vi "Micro-PL v10.6.4.vi"() -> ()   [LabVIEW 2010]
uses:
  drivers/Oxford ITC/ITCAPPS.LLB/ITCSetup.ctl
  drivers/Oxford ITC/ITCSUBS.LLB/ITCIO.ctl
  drivers/Oxford ITC/BUSGEN.LLB/OxfordAddress.ctl
  drivers/Oxford ITC/ITCSUBS.LLB/ITCVersion.ctl
  subvi/NPC3SG/TypeDefs/NPC3SG Live Controls.ctl
  subvi/NPC3SG/TypeDefs/NPC3SG Current Values.ctl
  subvi/NPC3SG/TypeDefs/NPC3SG Set Positions.ctl
  subvi/ITC503/TypeDefs/ITC503 Settings.ctl
  subvi/ITC503/TypeDefs/ITC503 Current Values.ctl
  subvi/iHR550/TypeDefs/iHR Current Values.ctl
  subvi/iHR550/TypeDefs/iHR Settings.ctl
  subvi/Mapping/TypeDefs/Mapping Spectra Params.ctl
  <vilib>/Utility/miscctls.llb/LVBoundsTypeDef.ctl
  subvi/Symphony/TypeDefs/Symphony Area Format.ctl
  <vilib>/Utility/miscctls.llb/LVPointTypeDef.ctl
  subvi/Mapping/TypeDefs/Mapping Input Parameters v10.6.2.ctl
  subvi/Global Variables.vi
  <vilib>/Analysis/NI_AALBase.lvlib
panel:
  in  "Update Supersize":bool caption="iHR550 Force Init"
  out "Graph Supersize Ref":refnum<vi>
  out "Spectrum Raw PX":dbl[][](array[numeric])
  out "Image Raw":i32[][](array[numeric])
  in  "Wavelength Recalculate":bool
  out "CCD Error":errorcluster
  out "Firmware":string="V1.20 CCD_4000"
  out "CCD Gain Number":i32[](array[numeric])=[10, 11, 12, 13, 8, 2]
  out "CCD ADC Number":i32[](array[numeric])=[0, 1, 2, 3, 4]
  out "JYCCDLib.IJYCCDReqd":refnum<k7>
  out "Spectrum Raw WL":dbl[][](array[numeric])
  out "Mapping State Storage":bool
  out "Drive Copy Target":bool
  in  "CCD Shutter":bool caption="Shutter:"
  out "Measurement Running":bool
  out "ITC Running":bool
  out "Drive Running":bool
  out "CCD Running":bool
  out "Mono Running":bool
  in  "Exit":bool
  out "Mono Status":bool
  out "Drive Status":bool
  out "CCD Status":bool
  out "ITC Status":bool
  in  "Register":enum32{"Devices", "Acquisition / Mapping"}(tab)
  in  "Mono Calibration":path=path "C:/Users/WET-KORR/Desktop/Calibration Data/iHR550 Coefficients 210915.ini"
  in  "Mono Force Init":bool=TRUE caption="iHR550 Force Init"
  in  "Mono Connect":bool
  in  "Mono ID":string(combo)="iHR550" caption="Monochromator ID"
  in  "Drive Calibration":path=path "C:/Users/WET-KORR/Desktop/Calibration Data/NPC3SG Objective Calibration 220216.ini"
  out "Drive Current Values":T1 {"Drive Z Position" min=-273.0 max=300000.0 step=0.0001 format="%.3f"; "Drive Y Position" min=-273.0 max=300000.0 step=0.0001 format="%.3f"; "Drive X Position" min=-273.0 max=300000.0 step=0.0001 format="%.3f"}
  in  "Drive Connection":refnum<visa-resource-name>="COM6" caption="COM Port"
  in  "Drive Connect":bool
  out "CCD Temp Graph":dbl(graph)=-134.538067
  in  "CCD Gain":u16(ring)=1 caption="Gain Mode" items=["High Light", "Best Dynamic Range", "High Sensitivity"]
  in  "Image Mode":bool caption="Image Mode?"
  in  "CCD Names":u16(ring) caption="CCD ID" items=["Symphony II"]
  in  "CCD Connect":bool
  out "CCD Temperature":dbl caption="Temp. (K)" min=10.0 max=160.0 step=0.1 format="%.1f"
  out "CCD Pixel X":i32=2048 caption="X Pixels"
  out "CCD Pixel Y":i32=512 caption="Y Pixels"
  out "CCD Data Size":i32=2048 caption="Data Size"
  in  "CCD ADC":u16(ring) caption="ADC Frequency" items=["20 kHz       ", " 1 MHz       ", " 1 MHz Ultra ", "500 kHz Wrap"]
  in  "CCD Configure":bool
  in  "CCD Area":T2={"XStart"=1, "YStart"=1, "XStop"=2048, "YStop"=512, "XBin"=1, "YBin"=1}
  in  "Snapshot Folder":path=path "C:/Users/WET-KORR/Desktop/Screenshots"
  in  "Camera Name":string="HD USB Camera"
  out "CCD IDs":u16(ring) items=["CCD1"]
  out "ITC Current Values":T3 {"ITC503 Gradient" format="%.2f"; "ITC503 Setpoint" min=-273.0 max=300000.0 step=0.0001 format="%.1f"; "ITC503 I" format="%_1f"; "ITC503 P" format="%_1f"; "ITC503 Temperature" min=0.0 max=1645.0 step=1e-05 format="%.2f"; "ITC503 Heater" min=0.0 max=100.0 step=0.01 scale=0.0..100.0}
  in  "ITC Settings":T4={"ITC503 Set Setpoint"=0.0, "ITC503 Set Auto Heater"=TRUE, "ITC503 Set Auto PID"=TRUE, "P"=0.0, "I"=0.0, "D"=0.0} {"D" min=0.0 max=100.0 step=0.1 format="%.1f"; "I" min=0.0 max=100.0 step=0.1 format="%.1f"; "P" min=0.0 max=100.0 step=0.1 format="%.1f"; "ITC503 Set Setpoint" min=-273.0 max=300000.0 step=0.1 format="%.1f"}
  in  "ITC Configure":bool
  in  "ITC Connect":bool
  in  "ITC Selector":u16(ring) caption="Select Device" items=["ITC503s"]
  out "Mono Timing":u32 caption="Mono"
  out "Drive Timing":u32 caption="Drive"
  out "ITC Timing":u32 caption="ITC"
  out "CCD Timing":u32 caption="CCD"
  in  "Graph Maximize":bool
  in  "Spectrum Axis":u16(ring)=1 caption="Axis" items=["Pixel", "Wavelength", "Energy"]
  in  "Spectrum Autosave":bool caption="iHR550 Force Init"
  in  "CCD Preview":bool
  in  "CCD Acquire":bool
  in  "Spectrum Settings":T5={"Integration Time"=1.0, "Repetitions"=1, "Mapping Spectra"=TRUE} caption="Mapping Spectra Settings" {"Repetitions" min=1 max=100 step=1; "Integration Time" min=0.1 max=6000.0 step=0.1 format="%.1f"}
  in  "CCD Current Rep.":string="0/0"
  out "Spectrum":cluster{dbl[], dbl[]}[](graph)
  in  "Spectrum Noise":i64 caption="Noise Level"
  in  "Spectrum Load":bool
  in  "Spectrum Save":bool
  out "Image":dbl[][](graph)
  in  "Video Show":bool
  in  "Drive GoTo":bool caption="Objective Move Abs."
  in  "Drive New Positions":T6 {"Drive X Set" min=10.0 max=160.0 step=0.1 format="%.3f"; "Drive Z Set" min=10.0 max=160.0 step=0.1 format="%.3f"; "Drive Y Set" min=10.0 max=160.0 step=0.1 format="%.3f"}
  out "Drive Live Current Values":T1 {"Drive Z Position" min=-273.0 max=300000.0 step=0.0001 format="%.3f"; "Drive Y Position" min=-273.0 max=300000.0 step=0.0001 format="%.3f"; "Drive X Position" min=-273.0 max=300000.0 step=0.0001 format="%.3f"}
  in  "Drive Live Controls":T7={"Snapshot"=FALSE, "Move Step"=0.5, "Move Home"=FALSE, "Move Down"=FALSE, "Move Up"=FALSE, "Move Left"=FALSE, "Move Right"=FALSE, "Move Out"=FALSE, "Move In"=FALSE} {"Move Step" min=0.0 max=30.0 step=0.1 format="%.3f"}
  in  "Mapping Start":bool
  in  "Mono Configure":bool
  in  "Mono Settings":T8={"iHR550 Set Exit Mirror"=2, "iHR550 Set Side Exit"=0.0, "iHR550 Set Front Entrance"=0.0, "iHR550 Set Wavelength"=897.9988, "iHR550 Set Grating"=0, "iHR550 Set Grating Switch"=FALSE, "iHR550 Set Wavelength Switch"=FALSE, "iHR550 Set Mirror Switch"=FALSE, "iHR550 Set Slits Switch"=FALSE} {"iHR550 Set Grating" items=["1800"=1, "600"=2, "150"=3]; "iHR550 Set Wavelength" min=0.0 max=1500.0 step=1.0; "iHR550 Set Side Exit" min=0.0 max=2000.0 step=1.0; "iHR550 Set Exit Mirror" items=["Front"=2, "Side"=3]}
  out "Mono Current Values":T9={"iHR 550 Front Entrance"=0.0, "iHR550 Side Exit"=0.0, "iHR550 Wavelength"=897.9988, "iHR550 Exit Mirror"=2, "iHR550 Grating"="1", "Grating Index"=1} {"iHR550 Exit Mirror" items=["EntranceMirror", "ExitMirror", "Front", "Side"]}
  out "ITC Temp Storage":dbl
  out "Runtime":u32
  out "ITC Gradient Time":i64
  out "ITC Read":bool
  out "CCD Read":bool
  out "Mono Read":bool
  out "Drive Read":bool
  out "Spectrum Properties":cluster{"Position":T10, "Plot Area Size":T10}={"Position"={"Width"=36, "Height"=367}, "Plot Area Size"={"Width"=496, "Height"=264}}
  in  "Auto Folder":path caption="Ausgewählter Pfad"
  out "Wavelengths (nm)":dbl[](array[numeric])
  out "iHR550 RefNum":refnum<k7> caption="Mono RefNum out"
  out "ITC Setup":T11={"Description"="", "IO Info"={"Address"={"Com Port"=1, "ISOBUS Address"=1, "GPIB Address"=24, "Communication"=enum."ISOBUS"}, "Version"=enum."ITC503", "Ch 1 dec places"=1, "Ch 2 dec places"=1, "Ch 3 dec places"=1, "Ch1 Name"="", "Ch2 Name"="", "Ch3 Name"=""}}
  # "Micro-PL Setup"
  # "Active"
  # "Active"
  # "ITC"
  # "iHR"
  # "Drive"
  # "CCD"
  # "Status"
  # "CCD"
  # "ITC"
  # "iHR"
  # "Drive"
  # "CCD"
  # "Monochromator"
  # "Objective Drive"
  # "Video"
  # "Cryostat"
  # "Timing"
  # "CCD"
  # "Acquisition"
  # "Drive Control"
  # "XY"
  # "Z"
  # "Mapping"
  # "Launch the Spectral Mapping VI and Raman Live Tool Set in a new window."
  # "Monochromator"
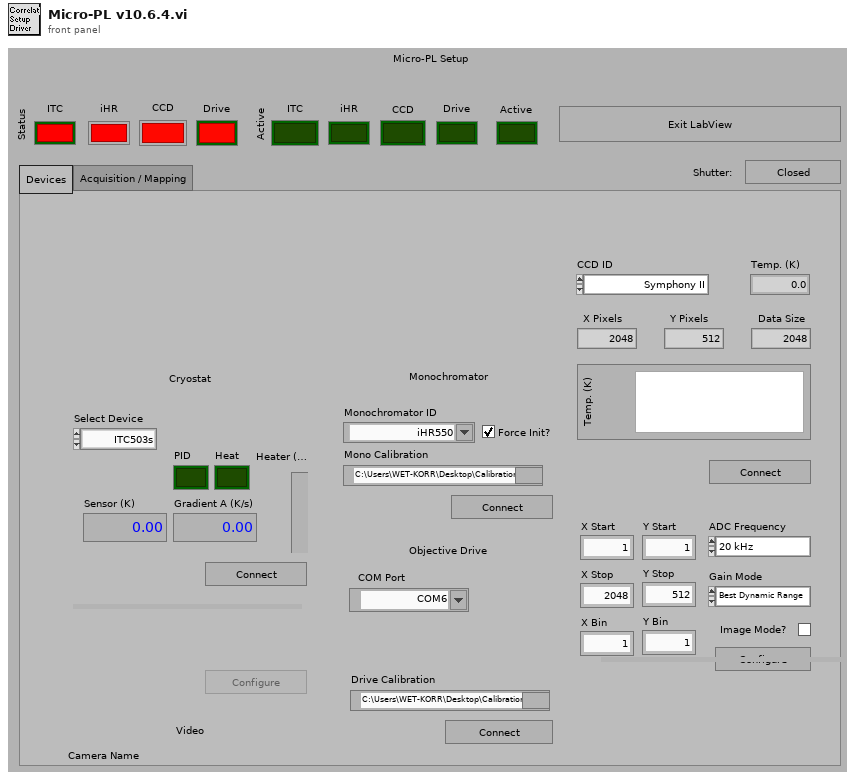
[diagram p1: front panel]
types:
  T1 = typedef "NPC3SG Current Values.ctl" = cluster{"Drive X Position":dbl, "Drive Y Position":dbl, "Drive Z Position":dbl}
  T2 = typedef "Symphony Area Format.ctl" = cluster{"XStart":i32, "YStart":i32, "XStop":i32, "YStop":i32, "XBin":i32, "YBin":i32}
  T3 = typedef "ITC503 Current Values.ctl" = cluster{"ITC503 Heater":dbl, "ITC503 Temperature":dbl, "ITC503 P":dbl, "ITC503 I":dbl, "ITC503 D":dbl, "ITC503 Setpoint":dbl, "ITC503 Gradient":dbl, "ITC503 Heater Auto":bool, "ITC503 PID Auto":bool}
  T4 = typedef "ITC503 Settings.ctl" = cluster{"ITC503 Set Setpoint":dbl, "ITC503 Set Auto Heater":bool, "ITC503 Set Auto PID":bool, "P":dbl, "I":dbl, "D":dbl}
  T5 = typedef "Mapping Spectra Params.ctl" = cluster{"Integration Time":dbl, "Repetitions":u16, "Mapping Spectra":bool}
  T6 = typedef "NPC3SG Set Positions.ctl" = cluster{"Drive X Set":dbl, "Drive Y Set":dbl, "Drive Z Set":dbl}
  T7 = typedef "NPC3SG Live Controls.ctl" = cluster{"Snapshot":bool, "Move Step":dbl, "Move Home":bool, "Move Down":bool, "Move Up":bool, "Move Left":bool, "Move Right":bool, "Move Out":bool, "Move In":bool}
  T8 = typedef "iHR Settings.ctl" = cluster{"iHR550 Set Exit Mirror":u16, "iHR550 Set Side Exit":dbl, "iHR550 Set Front Entrance":dbl, "iHR550 Set Wavelength":dbl, "iHR550 Set Grating":u16, "iHR550 Set Grating Switch":bool, "iHR550 Set Wavelength Switch":bool, "iHR550 Set Mirror Switch":bool, "iHR550 Set Slits Switch":bool}
  T9 = typedef "iHR Current Values.ctl" = cluster{"iHR 550 Front Entrance":dbl, "iHR550 Side Exit":dbl, "iHR550 Wavelength":dbl, "iHR550 Exit Mirror":i32, "iHR550 Grating":string, "Grating Index":i32}
  T10 = typedef "LVBoundsTypeDef.ctl" = cluster{"Width":u32, "Height":u32}
  T11 = typedef "ITCSetup.ctl" = cluster{"Description":string, "IO Info":T12}
  T12 = typedef "ITCIO.ctl" = cluster{"Address":T13, "Version":T14, "Ch 1 dec places":i16, "Ch 2 dec places":i16, "Ch 3 dec places":i16, "Ch1 Name":string, "Ch2 Name":string, "Ch3 Name":string}
  T13 = typedef "OxfordAddress.ctl" = cluster{"Com Port":i32, "ISOBUS Address":i32, "GPIB Address":i16, "Communication":enum16{"RS232", "ISOBUS", "GPIB", "Gateway"}}
  T14 = typedef "ITCVersion.ctl" = enum16{"ITC502", "ITC503", "ITC601"}
  T15 = enum8{"Enabled", "Disabled", "Disabled and Grayed Out"}
  T16 = typedef "LVPointTypeDef.ctl" = cluster{"Horizontal":i16, "Vertical":i16}
  T17 = enum16{"fire", "rainbow", "gray", "inverse gray", "ice", "original"}
  T18 = enum32{"Invalid", "Standard", "Closed", "Hidden", "Minimized", "Maximized"}
  T19 = typedef "Mapping Input Parameters v10.6.2.ctl" = cluster{"Drive Connection Port":refnum<visa-resource-name>, "ITC503 Current Values":T3, "Wavelengths (nm)":dbl[], "Drive Current Values":T1, "iHR Current Values":T9, "Spectra Settings":T5, "CCD3500 Temperature":dbl, "Simulate Drive":bool, "Simulate Spectra":bool, "JYCCDLib.IJYCCDReqd":refnum<k7>, "CCD Area":T2, "CCD Gain":u16, "CCD ADC":u16, "Drive Calibration":path}
  T20 = cluster{"Intensities":dbl[], "Wavelengths":dbl[]}[]
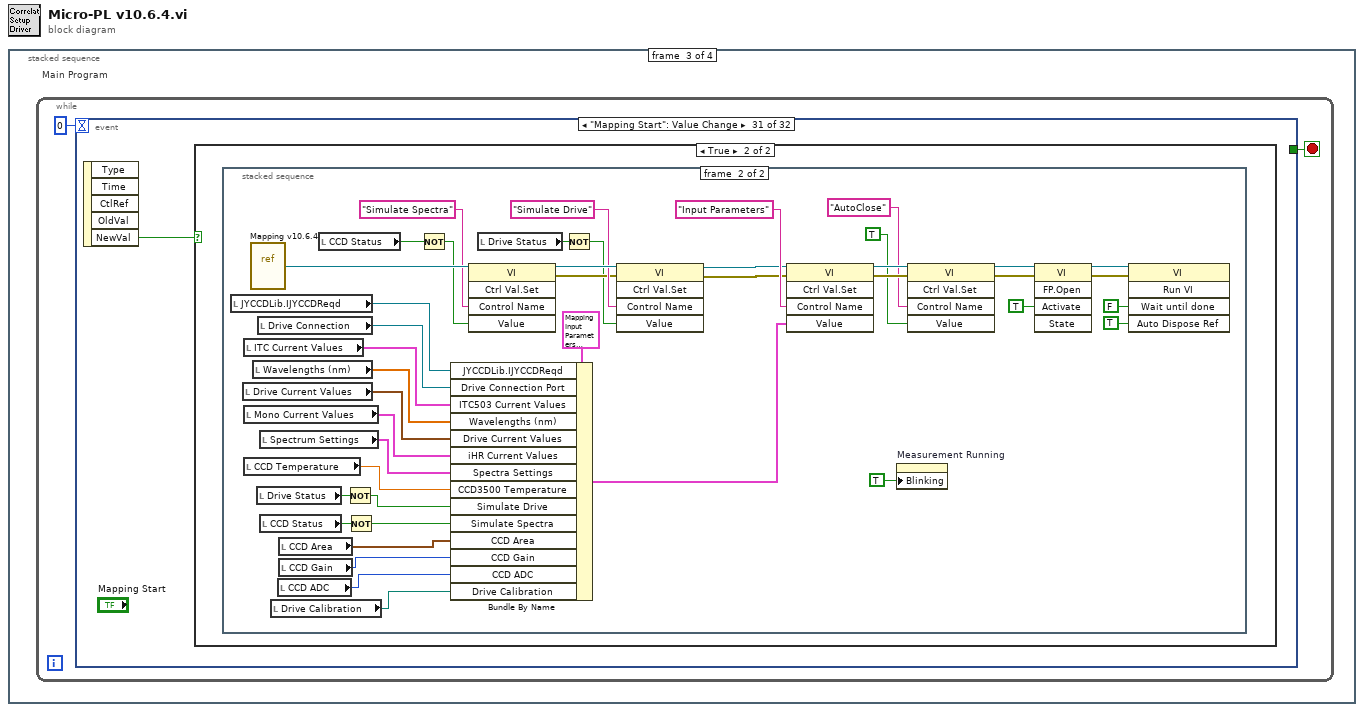
[diagram p0: block diagram]
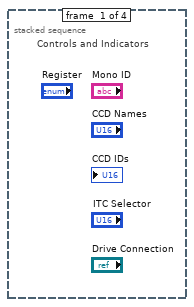
[diagram p2: hidden frame]
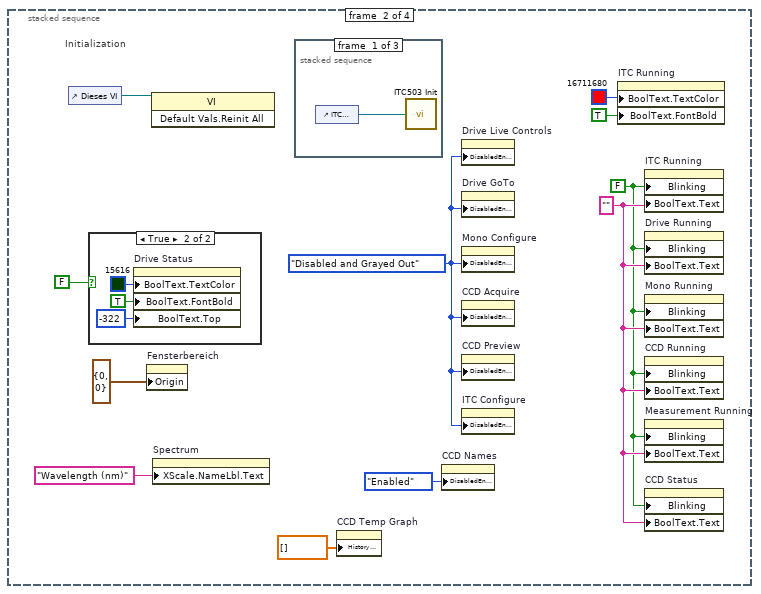
[diagram p3: hidden frame]
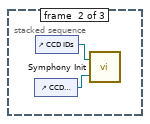
[diagram p4: hidden frame]
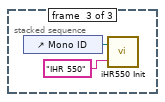
[diagram p5: hidden frame]
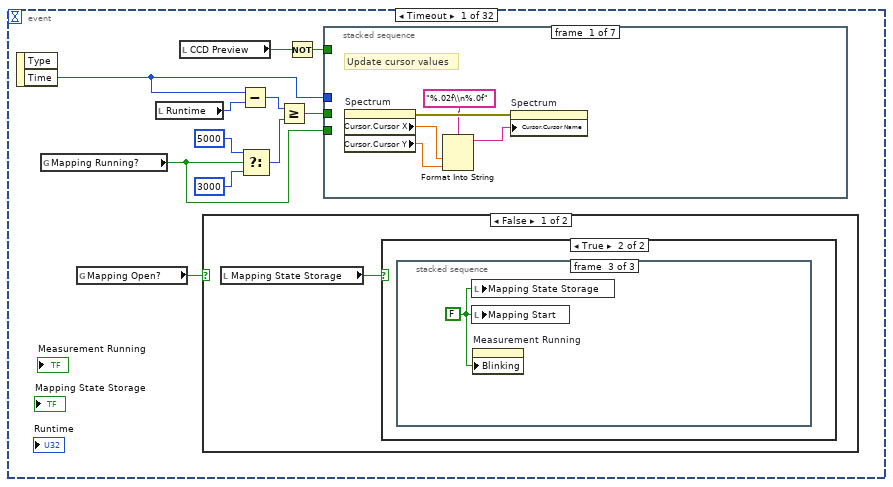
[diagram p7: hidden frame]
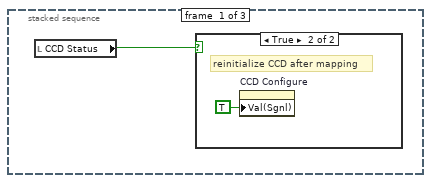
[diagram p9: hidden frame]
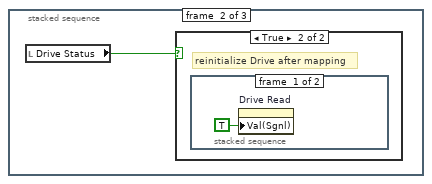
[diagram p11: hidden frame]
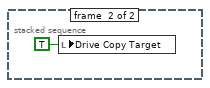
[diagram p13: hidden frame]
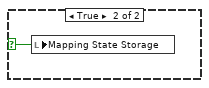
[diagram p14: hidden frame]
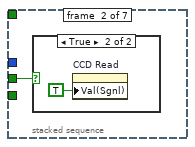
[diagram p15: hidden frame]
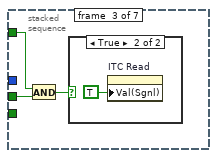
[diagram p17: hidden frame]
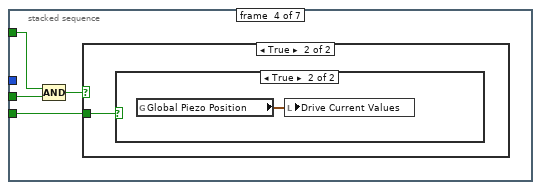
[diagram p19: hidden frame]
diagram:
  n1 = stacked-sequence {
    frame #0 {
      # "Controls and Indicators"
    }
    frame #1 {
      w3 = "" ("Boolean Text.Text")
      w2 = FALSE ("Blinking")
      w8 = T15."Disabled and Grayed Out" ("Deaktiviert")
      # "Initialization"
      n2 = control-ref of="Dieses VI"() -> (w11:refnum<vi>)
      n3 = case shown="True" FALSE {
        frame False {
        }
        frame True {
          n4 = property on="Drive Status" class="Bool (strict)"("BoolText.TextColor"=u32 15616, "BoolText.FontBold"=TRUE ("Boolescher Text.Schriftart:Fett"), "BoolText.Top"=-322 ("Boolescher Text.Position:Oben")) -> ()  [unwired: 2 in, 2 out]
        }
      }
      n5 = property on="Fensterbereich" class="Pane"("Origin"=T16 {"Horizontal"=0, "Vertical"=0}) -> ()  [unwired: 2 in, 2 out]
      n6 = invoke class="VI" method="Default Vals.Reinit All"(reference=w11) -> ()  [unwired: 2 in, 3 out]
      n7 = property on="Spectrum" class="XYGraph (strict)"("XScale.NameLbl.Text"="Wavelength (nm)" ("X Scale.Name Label.Text")) -> ()  [unwired: 2 in, 2 out]
      n8 = stacked-sequence {
        frame #0 {
          n9 = control-ref of="ITC Selector"() -> (w12:refnum<vi>)
          n10 = call "ITC503 Init.vi"("ITC Selector"=w12) -> ()  [unwired: 1 in]
        }
        frame #1 {
          n11 = control-ref of="CCD Names"() -> (w13:refnum<vi>)
          n12 = control-ref of="CCD IDs"() -> (w14:refnum<vi>)
          n13 = call "Symphony Init.vi"("Device Names"=w13, "Device IDs"=w14) -> ()
        }
        frame #2 {
          n14 = control-ref of="Mono ID"() -> (w16:refnum<vi>)
          n15 = call "iHR550 Init.vi"("Mono ID"=w16, "Target ID"="IHR 550") -> ()  [unwired: 1 in]
        }
      }
      n16 = property on="CCD Temp Graph" class="WFChart (strict)"("History Data"=dbl[] []) -> ()  [unwired: 2 in, 2 out]
      n17 = property on="CCD Names" class="Ring (strict)"("DisabledEnum"=T15."Enabled" ("Disabled")) -> ()  [unwired: 2 in, 2 out]
      n18 = property on="Drive Live Controls" class="Clust (strict)"("DisabledEnum"=w8) -> ()  [unwired: 2 in, 2 out]
      n19 = property on="Drive GoTo" class="Bool (strict)"("DisabledEnum"=w8) -> ()  [unwired: 2 in, 2 out]
      n20 = property on="Mono Configure" class="Bool (strict)"("DisabledEnum"=w8) -> ()  [unwired: 2 in, 2 out]
      n21 = property on="CCD Acquire" class="Bool (strict)"("DisabledEnum"=w8) -> ()  [unwired: 2 in, 2 out]
      n22 = property on="CCD Preview" class="Bool (strict)"("DisabledEnum"=w8) -> ()  [unwired: 2 in, 2 out]
      n23 = property on="ITC Configure" class="Bool (strict)"("DisabledEnum"=w8) -> ()  [unwired: 2 in, 2 out]
      n24 = property on="ITC Running" class="Bool (strict)"("BoolText.TextColor"=u32 16711680, "BoolText.FontBold"=TRUE ("Boolean Text.Font:Bold")) -> ()  [unwired: 2 in, 2 out]
      n25 = property on="ITC Running" class="Bool (strict)"("Blinking"=w2, "BoolText.Text"=w3) -> ()  [unwired: 2 in, 2 out]
      n26 = property on="Drive Running" class="Bool (strict)"("Blinking"=w2, "BoolText.Text"=w3) -> ()  [unwired: 2 in, 2 out]
      n27 = property on="Mono Running" class="Bool (strict)"("Blinking"=w2, "BoolText.Text"=w3) -> ()  [unwired: 2 in, 2 out]
      n28 = property on="CCD Running" class="Bool (strict)"("Blinking"=w2, "BoolText.Text"=w3) -> ()  [unwired: 2 in, 2 out]
      n29 = property on="Measurement Running" class="Bool (strict)"("Blinking"=w2, "BoolText.Text"=w3) -> ()  [unwired: 2 in, 2 out]
      n30 = property on="CCD Status" class="Bool (strict)"("Blinking"=w2, "BoolText.Text"=w3) -> ()  [unwired: 2 in, 2 out]
    }
    frame #2 {
      # "Main Program"
      n31 = while "Main-Program" {
        stop <- w21 stop-if-true
        n32 = event shown="[30] \"Mapping Start\": Value Change" {
          selector: _ -> [_ _ _ _ _ _ _ _ _ _ _ _ _ _ _ _ _ _ _ _ _ _ _ _ _ _ _ _ _ _ _ _]
          dyn-events: _ -> [_ _ _ _ _ _ _ _ _ _ _ _ _ _ _ _ _ _ _ _ _ _ _ _ _ _ _ _ _ _ _ _]
          timeout: 0 -> [_ _ _ _ _ _ _ _ _ _ _ _ _ _ _ _ _ _ _ _ _ _ _ _ _ _ _ _ _ _ _ _]
          tunnel: [_ w70 _ _ _ _ _ _ _ _ _ _ _ _ _ _ _ _ _ _ _ _ _ _ _ _ _ _ _ _ _ _] -> w21
          event Timeout {
            n33 = event-data() -> ("Time"=w28:u32)  [unwired: 1 in, 1 out]
            n34 = global read "Global Variables.vi" "Mapping Running?"() -> (w23:bool)
            n35 = global read "Global Variables.vi" "Mapping Open?"() -> (w22:bool)
            n36 = local read "Runtime"() -> (w27:u32)
            n37 = local read "CCD Preview"() -> (w30:bool)
            n38 = case shown="False" w22 {
              selector: w22 -> [_ w40]
              frame False {
                n39 = local read "Mapping State Storage"() -> (w33:bool)
                n40 = case shown="True" w33 {
                  frame False {
                  }
                  frame True {
                    n41 = stacked-sequence {
                      frame #0 {
                        n42 = local read "CCD Status"() -> (w34:bool)
                        n43 = case shown="True" w34 {
                          frame False {
                          }
                          frame True {
                            # "reinitialize CCD after mapping"
                            n44 = property on="CCD Configure" class="Bool (strict)"("Val(Sgnl)"=TRUE ("Value (Signaling)")) -> ()  [unwired: 2 in, 2 out]
                          }
                        }
                      }
                      frame #1 {
                        n45 = local read "Drive Status"() -> (w36:bool)
                        n46 = case shown="True" w36 {
                          frame False {
                          }
                          frame True {
                            # "reinitialize Drive after mapping"
                            n47 = stacked-sequence {
                              frame #0 {
                                n48 = property on="Drive Read" class="Bool (strict)"("Val(Sgnl)"=TRUE ("Value (Signaling)")) -> ()  [unwired: 2 in, 2 out]
                              }
                              frame #1 {
                                n49 = local write "Drive Copy Target"(TRUE ("Copy Drive Target")) -> ()
                              }
                            }
                          }
                        }
                      }
                      frame #2 {
                        w39 = FALSE ("Mapping Start")
                        n50 = local write "Mapping State Storage"(w39) -> ()
                        n51 = local write "Mapping Start"(w39) -> ()
                        n52 = property on="Measurement Running" class="Bool (strict)"("Blinking"=w39) -> ()  [unwired: 2 in, 2 out]
                      }
                    }
                  }
                }
              }
              frame True {
                n53 = local write "Mapping State Storage"(w40) -> ()
              }
            }
            n54 = Subtract(x=w28, y=w27) -> (x-y=w31:u32)
            n55 = Select(t=u32 5000 ("y"), s=w23, f=u32 3000 ("y")) -> (s? t:f=w24:u32)
            n56 = Greater Or Equal?(x=w31, y=w24) -> (x >= y?=w32:bool)
            n57 = Not(x=w30) -> (.not. x?=w29:bool)
            n58 = stacked-sequence {
              tunnel: w32 -> [_ w46 w50 w55 w62 _ w67]
              tunnel: w28 -> [_ _ _ _ _ _ w68]
              tunnel: w29 -> [_ _ w49 w54 w61 w64 _]
              tunnel: w23 -> [_ _ _ w52 w59 _ _]
              frame #0 {
                # "Update cursor values"
                n59 = property on="Spectrum" class="XYGraph (strict)"() -> (error out=w45:errorcluster, "Cursor.Cursor X"=w44:dbl, "Cursor.Cursor Y"=w43:dbl)  [unwired: 2 in, 1 out]
                n60 = Format Into String(format string="%.02f\\n%.0f", w44, w43) -> (resulting string=w41:string)  [unwired: 2 in, 1 out]
                n61 = property on="Spectrum" class="XYGraph (strict)"(error in=w45, "Cursor.Cursor Name"=w41) -> ()  [unwired: 1 in, 2 out]
              }
              frame #1 {
                n62 = case shown="True" w46 {
                  frame False {
                  }
                  frame True {
                    n63 = property on="CCD Read" class="Bool (strict)"("Val(Sgnl)"=TRUE ("Value (Signaling)")) -> ()  [unwired: 2 in, 2 out]
                  }
                }
              }
              frame #2 {
                n64 = And(x=w49, y=w50) -> (x .and. y?=w48:bool)
                n65 = case shown="True" w48 {
                  frame False {
                  }
                  frame True {
                    n66 = property on="ITC Read" class="Bool (strict)"("Val(Sgnl)"=TRUE ("Value (Signaling)")) -> ()  [unwired: 2 in, 2 out]
                  }
                }
              }
              frame #3 {
                n67 = Compound Arithmetic op=AND(w54, w55) -> (w53:bool)
                n68 = case shown="True" w53 {
                  tunnel: w52 -> [_ w56]
                  frame False {
                  }
                  frame True {
                    n69 = case shown="True" w56 {
                      frame False {
                        n70 = property on="Drive Read" class="Bool (strict)"("Val(Sgnl)"=TRUE ("Value (Signaling)")) -> ()  [unwired: 2 in, 2 out]
                      }
                      frame True {
                        n71 = global read "Global Variables.vi" "Global Piezo Position"() -> (w58:T1)
                        n72 = local write "Drive Current Values"(w58) -> ()
                      }
                    }
                  }
                }
              }
              frame #4 {
                n73 = Compound Arithmetic op=AND(w61, w62, w59) -> (w60:bool)
                n74 = case shown="True" w60 {
                  frame False {
                  }
                  frame True {
                    n75 = property on="Mono Read" class="Bool (strict)"("Val(Sgnl)"=TRUE ("Value (Signaling)")) -> ()  [unwired: 2 in, 2 out]
                  }
                }
              }
              frame #5 {
                n76 = case shown="False" w64 {
                  frame False {
                    n77 = flat-sequence {
                      frame #0 {
                        w65 = u32 50  # CCD buffer
                        n78 = Wait (ms)(milliseconds to wait=w65) -> ()  [unwired: 1 out]
                      }
                      frame #1 {
                        n79 = property on="CCD Acquire" class="Bool (strict)"("Val(Sgnl)"=TRUE ("Wert (signalisierend)")) -> ()  [unwired: 2 in, 2 out]
                      }
                    }
                  }
                  frame True {
                  }
                }
              }
              frame #6 {
                # "Set runtime counter"
                n80 = case shown="True" w67 {
                  tunnel: w68 -> [_ w69]
                  frame False {
                  }
                  frame True {
                    n81 = local write "Runtime"(w69) -> ()
                  }
                }
              }
            }
          }
          event "Exit": Value Change {
            n82 = event-data() -> ("NewVal"=w70:bool)  [unwired: 1 in, 4 out]
            n83 = stacked-sequence {
              frame #0 {
                n84 = local read "CCD Status"() -> (w71:bool)
                n85 = case shown="True" w71 {
                  frame False {
                  }
                  frame True {
                    n86 = local read "JYCCDLib.IJYCCDReqd"() -> (w72:refnum<k7>)
                    n87 = Close Reference(reference=w72) -> ()  [unwired: 1 in, 1 out]
                  }
                }
              }
              frame #1 {
                n88 = local read "Drive Status"() -> (w73:bool)
                n89 = case shown="True" w73 {
                  frame False {
                  }
                  frame True {
                    n90 = local read "Drive Connection"() -> (w74:refnum<visa-resource-name>)
                    n91 = call "NPC3SG Close.vi"("Drive Visa Name"=w74) -> ()  [unwired: 4 in]
                  }
                }
              }
            }
          }
          event "Mono Connect": Value Change {
            n92 = event-data() -> ("NewVal"=w75:bool)  [unwired: 1 in, 4 out]
            n93 = stacked-sequence {
              tunnel: w75 -> [_ w78 _]
              frame #0 {
                n94 = property on="Mono Running" class="Bool (strict)"("Blinking"=TRUE ("Blinkend")) -> ()  [unwired: 2 in, 2 out]
              }
              frame #1 {
                n95 = case shown="True" w78 {
                  selector: w78 -> [w82 _]
                  tunnel: [w82 w95] -> w77
                  frame False {
                    # "disconnect"
                  }
                  frame True {
                    # "connect"
                    n96 = local read "Mono Force Init"() -> (w93:bool)
                    n97 = control-ref of="iHR550 Set Grating"() -> (w94:refnum<vi>)
                    n98 = local read "Mono Calibration"() -> (w83:path)
                    n99 = local read "Mono ID"() -> (w96:string)
                    n100 = call "iHR550 Connect.vi"("Force\nInitialization"=w93, "Grating Selector"=w94, "Mono ID"=w96) -> ("Initialized"=w95:bool, "iHR550 RefNum"=w92:refnum<k7>)  [unwired: 2 in, 4 out]
                    n101 = local write "iHR550 RefNum"(w92) -> ()
                    n102 = call "iHR550 Read Values v10.6.2.vi"("Mono Calibration"=w83, "JYMONOLib.IJYMonoReqd"=w92) -> ("iHR Current Values"=w84:T9)  [unwired: 1 in]
                    n103 = Unbundle By Name(w84) -> ("iHR 550 Front Entrance"=w90:dbl, "iHR550 Side Exit"=w89:dbl, "iHR550 Wavelength"=w88:dbl, "iHR550 Exit Mirror"=w87:i32, "Grating Index"=w85:i32)
                    n104 = local write "Mono Current Values"(w84) -> ()
                    n105 = Bundle By Name(cluster=T8 {"iHR550 Set Exit Mirror"=0, "iHR550 Set Side Exit"=0.0, "iHR550 Set Front Entrance"=0.0, "iHR550 Set Wavelength"=0.0, "iHR550 Set Grating"=0, "iHR550 Set Grating Switch"=FALSE, "iHR550 Set Wavelength Switch"=FALSE, "iHR550 Set Mirror Switch"=FALSE, "iHR550 Set Slits Switch"=FALSE} ("iHR Settings"), "iHR550 Set Front Entrance"=w90, "iHR550 Set Side Exit"=w89, "iHR550 Set Wavelength"=w88, "iHR550 Set Exit Mirror"=w87, "iHR550 Set Grating"=w85) -> (w86:T8)
                    n106 = local write "Mono Settings"(w86) -> ()
                  }
                }
                n107 = case shown="False" w77 {
                  tunnel: [T15."Disabled and Grayed Out" ("Deaktiviert") T15."Enabled" ("Deaktiviert")] -> w79
                  frame False {
                  }
                  frame True {
                  }
                }
                n108 = local write "Mono Connect"(w77) -> ()
                n109 = local write "Mono Status"(w77) -> ()
                n110 = property on="Mono Configure" class="Bool (strict)"("DisabledEnum"=w79) -> ()  [unwired: 2 in, 2 out]
              }
              frame #2 {
                w98 = TRUE ("Wert (signalisierend)")
                w97 = FALSE ("Blinkend")
                n111 = local write "Mono Force Init"(w97) -> ()
                n112 = property on="Mono Running" class="Bool (strict)"("Blinking"=w97) -> ()  [unwired: 2 in, 2 out]
                n113 = property on="Mono Read" class="Bool (strict)"("Val(Sgnl)"=w98) -> ()  [unwired: 2 in, 2 out]
                n114 = property on="Wavelength Recalculate" class="Bool (strict)"("Val(Sgnl)"=w98) -> ()  [unwired: 2 in, 2 out]
              }
            }
          }
          event "Mono Read": Value Change {
            n115 = event-data() -> ("NewVal"=w102:bool)  [unwired: 1 in, 4 out]
            n116 = local read "Mono Status"() -> (w101:bool)
            n117 = And(x=w101, y=w102) -> (x .and. y?=w100:bool)
            n118 = case shown="True" w100 {
              tunnel: [u32 0 w104] -> w99
              frame False {
              }
              frame True {
                n119 = stacked-sequence {
                  seq-local: [w105 _ _] -> [_ _ w109]
                  tunnel: [_ _ w110] -> w104
                  frame #0 {
                    n120 = Tick Count (ms)() -> (millisecond timer value=w105:u32)
                  }
                  frame #1 {
                    n121 = local read "Mono Calibration"() -> (w106:path)
                    n122 = local read "iHR550 RefNum"() -> (w108:refnum<k7>)
                    n123 = call "iHR550 Read Values v10.6.2.vi"("Mono Calibration"=w106, "JYMONOLib.IJYMonoReqd"=w108) -> ("iHR Current Values"=w107:T9)  [unwired: 1 in]
                    n124 = local write "Mono Current Values"(w107) -> ()
                    n125 = global write "Global Variables.vi" "Global iHR Values"(w107) -> ()
                  }
                  frame #2 {
                    n126 = Tick Count (ms)() -> (millisecond timer value=w111:u32)
                    n127 = Subtract(x=w111, y=w109) -> (x-y=w110:u32)
                  }
                }
              }
            }
            "Mono Timing" <- w99
          }
          event "Mono Configure": Value Change {
            n128 = event-data() -> ("NewVal"=w112:bool)  [unwired: 1 in, 4 out]
            n129 = stacked-sequence {
              tunnel: w112 -> [_ w114 _]
              frame #0 {
                n130 = property on="Mono Running" class="Bool (strict)"("Blinking"=TRUE ("Blinkend")) -> ()  [unwired: 2 in, 2 out]
              }
              frame #1 {
                n131 = local read "Mono Status"() -> (w116:bool)
                n132 = And(x=w116, y=w114) -> (x .and. y?=w115:bool)
                n133 = case shown="True" w115 {
                  frame False {
                  }
                  frame True {
                    n134 = stacked-sequence {
                      frame #0 {
                        w121 = u16 2 items=["Front"=2, "Side"=3] ("Entrance Mirror")
                        n135 = local read "iHR550 RefNum"() -> (w118:refnum<k7>)
                        n136 = local read "Mono Calibration"() -> (w117:path)
                        n137 = local read "Mono Settings"() -> (w119:T8)
                        n138 = call "iHR550 Set Values v10.6.2.vi"("Refnum out"=w118, "Entrance Mirror"=w121, "Target\nSide Entrance"=0.0 ("Target\nSide Entrance"), "iHR Settings"=w119, "Mono Calibration"=w117) -> ()  [unwired: 10 in, 1 out]
                      }
                      frame #1 {
                        n139 = property on="Mono Read" class="Bool (strict)"("Val(Sgnl)"=TRUE ("Value (Signaling)")) -> ()  [unwired: 2 in, 2 out]
                      }
                      frame #2 {
                        n140 = property on="Wavelength Recalculate" class="Bool (strict)"("Val(Sgnl)"=TRUE ("Value (Signaling)")) -> ()  [unwired: 2 in, 2 out]
                      }
                    }
                  }
                }
              }
              frame #2 {
                w125 = FALSE ("Blinkend")
                n141 = property on="Mono Read" class="Bool (strict)"("Val(Sgnl)"=TRUE ("Wert (signalisierend)")) -> ()  [unwired: 2 in, 2 out]
                n142 = property on="Mono Running" class="Bool (strict)"("Blinking"=w125) -> ()  [unwired: 2 in, 2 out]
                n143 = local write "Mono Configure"(w125) -> ()
              }
            }
          }
          event "CCD Connect": Value Change {
            n144 = event-data() -> ("NewVal"=w126:bool)  [unwired: 1 in, 4 out]
            n145 = stacked-sequence {
              tunnel: w126 -> [_ w130 _]
              frame #0 {
                n146 = local read "CCD Names"() -> (w127:u16)
                n147 = property on="CCD Running" class="Bool (strict)"("Blinking"=TRUE ("Blinkend")) -> ()  [unwired: 2 in, 2 out]
                n148 = local write "CCD IDs"(w127) -> ()
              }
              frame #1 {
                n149 = case shown="False" w130 {
                  selector: w130 -> [w141 _]
                  tunnel: [w141 w150] -> w132
                  frame False {
                    # "disconnect"
                    n150 = local read "JYCCDLib.IJYCCDReqd"() -> (w140:refnum<k7>)
                    n151 = property on="CCD Status" class="Bool (strict)"("Blinking"=FALSE, "BoolText.Text"="" ("Boolean Text.Text")) -> ()  [unwired: 2 in, 2 out]
                    n152 = local read "CCD Error"() -> (w139:errorcluster)
                    n153 = Close Reference(reference=w140, error in (no error)=w139) -> ()  [unwired: 1 out]
                  }
                  frame True {
                    # "connect"
                    n154 = local read "CCD IDs"() -> (w155:u16)
                    n155 = property on="CCD IDs" class="Ring (strict)"() -> ("Chaînes []"=w154:string[])  [unwired: 2 in, 2 out]
                    n156 = Index Array(array=w154, index=w155) -> (element=w156:string)
                    n157 = call "Initialize CCD.vi"("Unique id:"=w156) -> ("activeYPixels"=w143:i32, "JYCCDLib.IJYCCDReqd"=w157:refnum<k7>, "activeXPixels"=w145:i32, "sortie d'erreur"=w158:errorcluster, "FirmwareVersion"=→"Firmware":string)  [unwired: 3 out]
                    "CCD Pixel X" <- w145
                    "CCD Pixel Y" <- w143
                    n158 = call "Trigger - Disable.vi"("Error In"=w158, "JYCCDLib.IJYCCDReqd"=w157) -> ("Error Out"=w152:errorcluster, "JYCCDLib.IJYCCDReqd"=w163:refnum<k7>)  [unwired: 4 out]
                    n159 = local read "CCD Area"() -> (w149:T2)
                    n160 = Bundle By Name(cluster=w149, "XStart"=1, "XStop"=w145, "YStart"=1, "YStop"=w143, "XBin"=1, "YBin"=1) -> (w148:T2)
                    n161 = local write "CCD Error"(w152) -> ()
                    n162 = call "Init ADC & Gain.vi"("JYCCDLib.IJYCCDReqd"=w163, "input error"=w152) -> ("ADC Number"=w159:i32[], "ADC description"=w161:string[], "Gain Number"=w160:i32[], "Gain description"=w162:string[])
                    n163 = local write "JYCCDLib.IJYCCDReqd"(w163) -> ()
                    n164 = local write "CCD Area"(w148) -> ()
                    n165 = local write "CCD ADC Number"(w159) -> ()
                    n166 = local write "CCD Gain Number"(w160) -> ()
                    n167 = property on="CCD ADC" class="Ring (strict)"("Chaînes []"=w161) -> ()  [unwired: 2 in, 2 out]
                    n168 = property on="CCD Gain" class="Ring (strict)"("Chaînes []"=w162) -> ()  [unwired: 2 in, 2 out]
                    n169 = call <vilib>:"Simple Error Handler.vi"("error in (no error)"=w152) -> ("error?"=w151:bool)  [unwired: 4 in, 4 out]
                    n170 = Not(x=w151) -> (.not. x?=w150:bool)
                  }
                }
                n171 = case shown="False" w132 {
                  tunnel: [T15."Disabled and Grayed Out" ("Deaktiviert") T15."Enabled" ("Deaktiviert")] -> w131
                  tunnel: [T15."Enabled" ("Deaktiviert") T15."Disabled and Grayed Out" ("Deaktiviert")] -> w129
                  frame False {
                  }
                  frame True {
                  }
                }
                n172 = property on="CCD Status" class="Bool (strict)"("BoolText.Visible"=w132) -> ()  [unwired: 2 in, 2 out]
                n173 = local write "CCD Connect"(w132) -> ()
                n174 = local write "CCD Status"(w132) -> ()
                n175 = property on="CCD Acquire" class="Bool (strict)"("DisabledEnum"=w131) -> ()  [unwired: 2 in, 2 out]
                n176 = property on="CCD Preview" class="Bool (strict)"("DisabledEnum"=w131) -> ()  [unwired: 2 in, 2 out]
                n177 = property on="CCD Names" class="Ring (strict)"("Désactivé"=w129) -> ()  [unwired: 2 in, 2 out]
                n178 = property on="CCD IDs" class="Ring (strict)"("Désactivé"=w129) -> ()  [unwired: 2 in, 2 out]
              }
              frame #2 {
                w164 = TRUE ("Wert (signalisierend)")
                n179 = property on="CCD Configure" class="Bool (strict)"("Val(Sgnl)"=w164) -> (error out=w165:errorcluster)  [unwired: 2 in, 1 out]
                n180 = property on="CCD Running" class="Bool (strict)"("Blinking"=FALSE ("Blinkend")) -> ()  [unwired: 2 in, 2 out]
                n181 = property on="CCD Read" class="Bool (strict)"(error in=w165, "Val(Sgnl)"=w164) -> ()  [unwired: 1 in, 2 out]
              }
            }
          }
          event "CCD Read": Value Change {
            n182 = event-data() -> ("NewVal"=w170:bool)  [unwired: 1 in, 4 out]
            n183 = local read "CCD Status"() -> (w169:bool)
            n184 = And(x=w169, y=w170) -> (x .and. y?=w168:bool)
            n185 = case shown="True" w168 {
              tunnel: [u32 0 w172] -> w167
              frame False {
              }
              frame True {
                n186 = stacked-sequence {
                  seq-local: [_ w174 _ _] -> [_ _ w182 _]
                  seq-local: [w173 _ _ _] -> [_ _ _ w193]
                  tunnel: [_ _ _ w194] -> w172
                  frame #0 {
                    n187 = Tick Count (ms)() -> (millisecond timer value=w173:u32)
                  }
                  frame #1 {
                    w175 = u16 1 items=["° Celsius", "Kelvin", "° Farenheit"] ("units")
                    n188 = local read "JYCCDLib.IJYCCDReqd"() -> (w178:refnum<k7>)
                    n189 = local read "CCD Error"() -> (w176:errorcluster)
                    n190 = call "read temperature.vi"("entrée d'erreur (pas d'erreur)"=w176, "units"=w175, "JYCCDLib.IJYCCDReqd"=w178) -> ("error out"=w177:errorcluster, "Current Temperature"=w174:dbl)
                    n191 = local write "CCD Temp Graph"(w174) -> ()
                    n192 = local write "CCD Error"(w177) -> ()
                    n193 = local write "CCD Temperature"(w174) -> ()
                  }
                  frame #2 {
                    n194 = Subtract(x=w182, y=140.0) -> (x-y=w179:dbl)
                    n195 = Absolute Value(x=w179) -> (abs(x)=w180:dbl)
                    n196 = Greater?(x=w180, y=1.0) -> (0:w184:bool)
                    n197 = case shown="False" w184 {
                      selector: w184 -> [w190 w192]
                      tunnel: [cluster{u32, u32}[] [{16713728, 16713728}, {6618880, 6618880}] ("Farben [4]") cluster{u32, u32}[] [{16713728, 16713728}] ("Farben [4]")] -> w185
                      tunnel: [w190 w192] -> w187
                      frame False {
                      }
                      frame True {
                      }
                    }
                    n198 = Number To Fractional String(number=w182, precision (6)=i16 1 ("Genauigkeit (6)")) -> (F-format string=w186:string)  [unwired: 2 in]
                    n199 = global write "Global Variables.vi" "Global CCD Temperature (C)"(w182) -> ()
                    n200 = property on="CCD Status" class="Bool (strict)"("Blinking"=w187, "BoolText.Text"=w186, "Colors [4]"=w185) -> ()  [unwired: 2 in, 2 out]
                  }
                  frame #3 {
                    n201 = Tick Count (ms)() -> (millisecond timer value=w195:u32)
                    n202 = Subtract(x=w195, y=w193) -> (x-y=w194:u32)
                  }
                }
              }
            }
            "CCD Timing" <- w167
          }
          event "CCD Configure": Value Change {
            n203 = event-data() -> ("NewVal"=w197:bool)  [unwired: 1 in, 4 out]
            n204 = local read "CCD Status"() -> (w198:bool)
            n205 = And(x=w198, y=w197) -> (x .and. y?=w196:bool)
            n206 = case shown="True" w196 {
              frame False {
              }
              frame True {
                n207 = stacked-sequence {
                  frame #0 {
                    n208 = local read "Spectrum Settings"() -> (w203:T5)
                    n209 = local read "CCD Gain Number"() -> (w212:i32[])
                    n210 = local read "CCD ADC Number"() -> (w210:i32[])
                    n211 = local read "JYCCDLib.IJYCCDReqd"() -> (w201:refnum<k7>)
                    n212 = local read "CCD ADC"() -> (w209:u16)
                    n213 = local read "CCD Gain"() -> (w211:u16)
                    n214 = Unbundle By Name(w203) -> ("Integration Time"=w202:dbl)
                    n215 = local read "Image Mode"() -> (w206:bool)
                    n216 = local read "CCD Error"() -> (w205:errorcluster)
                    n217 = local read "CCD Area"() -> (w200:T2)
                    n218 = Index Array(array=w210, index=w209) -> (element=w208:i32)
                    n219 = Index Array(array=w212, index=w211) -> (element=w207:i32)
                    n220 = call "Symphony Setup.vi"("JYCCDLib.IJYCCDReqd"=w201, "ADC"=w208, "Image Mode"=w206, "Integration (s)"=w202, "Symphony Area Format"=w200, "Error Input"=w205, "Gain"=w207) -> ("DataSize"=w199:i32, "Error Output"=w204:errorcluster)  [unwired: 7 in]
                    n221 = local write "CCD Error"(w204) -> ()
                    n222 = local write "CCD Data Size"(w199) -> ()
                  }
                  frame #1 {
                    n223 = property on="Wavelength Recalculate" class="Bool (strict)"("Val(Sgnl)"=TRUE ("Value (Signaling)")) -> ()  [unwired: 2 in, 2 out]
                    n224 = local write "CCD Configure"(FALSE ("CCD Configure")) -> ()
                    n225 = local read "Image Mode"() -> (w216:bool)
                    n226 = call "Image Intensity Color Tables.vi"("Map Selector"=T17."original") -> ("Color Map Array"=w214:u32[])  [unwired: 10 in]
                    n227 = Not(x=w216) -> (.not. x?=w215:bool)
                    n228 = property on="Image" class="IntGraph (strict)"("Visible"=w216, "Color Table"=w214) -> ()  [unwired: 2 in, 2 out]
                    n229 = property on="Spectrum" class="XYGraph (strict)"("Visible"=w215) -> ()  [unwired: 2 in, 2 out]
                    n230 = property on="Spectrum Load" class="Bool (strict)"("Visible"=w215) -> ()  [unwired: 2 in, 2 out]
                    n231 = property on="Spectrum Noise" class="DigNum (strict)"("Visible"=w215) -> ()  [unwired: 2 in, 2 out]
                    n232 = property on="CCD Current Rep." class="Str"("Visible"=w215) -> ()  [unwired: 2 in, 2 out]
                  }
                }
              }
            }
          }
          event Value Change {
            n233 = event-data() -> ()  [unwired: 1 in, 5 out]
            n234 = stacked-sequence {
              frame #0 {
                w232 = 1 ("y")
                n235 = local read "CCD Area"() -> (w230:T2)
                n236 = Unbundle By Name(w230) -> ("XBin"=w226:i32, "YBin"=w231:i32)
                n237 = Logarithm Base 2(1:w231) -> (0:w227:dbl)
                n238 = Logarithm Base 2(1:w226) -> (0:w223:dbl)
                n239 = Quotient & Remainder(x=w227, y=w232) -> (x-y*floor(x/y)=w228:dbl, floor(x/y)=w229:dbl)
                n240 = Quotient & Remainder(x=w223, y=w232) -> (x-y*floor(x/y)=w224:dbl, floor(x/y)=w225:dbl)
                n241 = Not Equal To 0?(x=w228) -> (x != 0?=w222:bool)
                n242 = Not Equal To 0?(x=w224) -> (x != 0?=w221:bool)
                n243 = Or(x=w221, y=w222) -> (x .or. y?=w220:bool)
                n244 = case shown="True" w222 {
                  tunnel: w229 -> [_ w237]
                  tunnel: w230 -> [_ w235]
                  frame False {
                  }
                  frame True {
                    n245 = Power Of 2(x=w237) -> (2^x=w236:dbl)
                    n246 = Bundle By Name(cluster=w235, "YBin"=w236) -> (w234:T2)
                    n247 = local write "CCD Area"(w234) -> ()
                  }
                }
                n248 = case shown="True" w221 {
                  tunnel: w225 -> [_ w241]
                  tunnel: w230 -> [_ w239]
                  frame False {
                  }
                  frame True {
                    n249 = Power Of 2(x=w241) -> (2^x=w240:dbl)
                    n250 = Bundle By Name(cluster=w239, "XBin"=w240) -> (w238:T2)
                    n251 = local write "CCD Area"(w238) -> ()
                  }
                }
                n252 = case shown="True" w220 {
                  tunnel: "Binning factor has been adjusted  (must be an exponent of 2)." ("message") -> [_ w233]
                  frame False {
                  }
                  frame True {
                    n253 = One Button Dialog(message=w233) -> ()  [unwired: 1 in, 1 out]
                  }
                }
              }
              frame #1 {
                w260 = "Could not adjust CCD area to fit binning size!" ("message")
                w261 = "CCD area has been adjusted to fit binning size." ("message")
                n254 = local read "CCD Area"() -> (w242:T2)
                n255 = Unbundle By Name(w242) -> ("XStop"=w249:i32, "XStart"=w250:i32, "XBin"=w247:i32)
                n256 = Unbundle By Name(w242) -> ("YStop"=w254:i32, "YStart"=w255:i32, "YBin"=w259:i32)
                n257 = Subtract(x=w249, y=w250) -> (x-y=w243:i32)
                n258 = Subtract(x=w254, y=w255) -> (x-y=w252:i32)
                n259 = Increment(x=w243) -> (x+1=w248:i32)
                n260 = Increment(x=w252) -> (x+1=w256:i32)
                n261 = Quotient & Remainder(x=w248, y=w247) -> (x-y*floor(x/y)=w244:i32, floor(x/y)=w246:i32)
                n262 = Quotient & Remainder(x=w256, y=w259) -> (x-y*floor(x/y)=w253:i32, floor(x/y)=w258:i32)
                n263 = Not Equal To 0?(x=w244) -> (x != 0?=w245:bool)
                n264 = Not Equal To 0?(x=w253) -> (x != 0?=w257:bool)
                n265 = case shown="True" w257 {
                  tunnel: w254 -> [_ w279]
                  tunnel: w255 -> [_ w278]
                  tunnel: w256 -> [_ w277]
                  tunnel: w258 -> [_ w276]
                  tunnel: w259 -> [_ w275]
                  tunnel: w260 -> [_ w269]
                  tunnel: w261 -> [_ w270]
                  tunnel: w242 -> [_ w274]
                  tunnel: ["" ("message") w271] -> w263
                  frame False {
                  }
                  frame True {
                    n266 = Multiply(x=w276, y=w275) -> (x*y=w281:i32)
                    n267 = Subtract(x=w277, y=w281) -> (x-y=w280:i32)
                    n268 = Add(x=w278, y=w280) -> (x+y=w273:i32)
                    n269 = Greater?(x=w279, y=w273) -> (0:w272:bool)
                    n270 = case shown="True" w272 {
                      tunnel: w274 -> [_ w286]
                      tunnel: w273 -> [_ w285]
                      tunnel: [w282 w283] -> w271
                      tunnel: w270 -> [_ w283]
                      tunnel: w269 -> [w282 _]
                      frame False {
                      }
                      frame True {
                        n271 = Bundle By Name(cluster=w286, "YStart"=w285) -> (w284:T2)
                        n272 = local write "CCD Area"(w284) -> ()
                      }
                    }
                  }
                }
                n273 = case shown="True" w245 {
                  tunnel: w246 -> [_ w301]
                  tunnel: w247 -> [_ w300]
                  tunnel: w248 -> [_ w294]
                  tunnel: w249 -> [_ w297]
                  tunnel: w250 -> [_ w295]
                  tunnel: w242 -> [_ w293]
                  tunnel: ["" ("message") w291] -> w264
                  tunnel: w261 -> [_ w290]
                  tunnel: w260 -> [_ w289]
                  frame False {
                  }
                  frame True {
                    n274 = Multiply(x=w301, y=w300) -> (x*y=w299:i32)
                    n275 = Subtract(x=w294, y=w299) -> (x-y=w296:i32)
                    n276 = Add(x=w295, y=w296) -> (x+y=w292:i32)
                    n277 = Greater?(x=w297, y=w292) -> (0:w298:bool)
                    n278 = case shown="True" w298 {
                      tunnel: w293 -> [_ w306]
                      tunnel: w292 -> [_ w304]
                      tunnel: [w302 w303] -> w291
                      tunnel: w290 -> [_ w303]
                      tunnel: w289 -> [w302 _]
                      frame False {
                      }
                      frame True {
                        n279 = Bundle By Name(cluster=w306, "XStart"=w304) -> (w305:T2)
                        n280 = local write "CCD Area"(w305) -> ()
                      }
                    }
                  }
                }
                n281 = Empty String/Path?(string/path=w264) -> (empty?=w262:bool)
                n282 = case shown="False" w262 {
                  tunnel: [w266 w267] -> w265
                  tunnel: w263 -> [_ w267]
                  tunnel: w264 -> [w266 _]
                  frame False {
                  }
                  frame True {
                  }
                }
                n283 = Empty String/Path?(string/path=w265) -> (empty?=w251:bool)
                n284 = case shown="False" w251 {
                  tunnel: w265 -> [w287 _]
                  frame False {
                    n285 = One Button Dialog(message=w287) -> ()  [unwired: 1 in, 1 out]
                  }
                  frame True {
                  }
                }
              }
            }
          }
          event "CCD Shutter": Value Change {
            n286 = event-data() -> ("NewVal"=w307:bool)  [unwired: 1 in, 4 out]
            n287 = local read "CCD Status"() -> (w308:bool)
            n288 = case shown="False" w308 {
              tunnel: w307 -> [_ w310]
              frame False {
              }
              frame True {
                n289 = local read "JYCCDLib.IJYCCDReqd"() -> (w312:refnum<k7>)
                n290 = local read "CCD Error"() -> (w311:errorcluster)
                n291 = call "Shutter Control.vi"("input error"=w311, "Shutter"=w310, "JYCCDLib.IJYCCDReqd"=w312) -> ("error out"=w313:errorcluster)  [unwired: 1 out]
                n292 = call <vilib>:"Simple Error Handler.vi"("error in (no error)"=w313) -> ("error?"=w309:bool)  [unwired: 4 in, 4 out]
                n293 = local write "CCD Error"(w313) -> ()
                n294 = case shown="True" w309 {
                  tunnel: w310 -> [_ w314]
                  frame False {
                  }
                  frame True {
                    n295 = Not(x=w314) -> (.not. x?=w315:bool)
                    n296 = local write "CCD Shutter"(w315) -> ()
                  }
                }
              }
            }
          }
          event "CCD Acquire": Value Change {
            n297 = event-data() -> ("NewVal"=w316:bool)  [unwired: 1 in, 4 out]
            n298 = case shown="True" w316 {
              frame False {
              }
              frame True {
                n299 = stacked-sequence {
                  frame #0 {
                    n300 = local read "JYCCDLib.IJYCCDReqd"() -> (w317:refnum<k7>)
                    n301 = local read "Image Mode"() -> (w321:bool)
                    n302 = local read "CCD Error"() -> (w318:errorcluster)
                    n303 = control-ref of="CCD Acquire"() -> (w319:refnum<vi>)
                    n304 = control-ref of="CCD Running"() -> (w320:refnum<vi>)
                    n305 = case shown="False" w321 {
                      tunnel: w320 -> [w325 w376]
                      tunnel: w319 -> [w324 w375]
                      tunnel: w318 -> [w323 w377]
                      tunnel: w317 -> [w322 w378]
                      frame False {
                        n306 = local read "CCD Preview"() -> (w326:bool)
                        n307 = local read "Spectrum Settings"() -> (w327:T5)
                        n308 = Unbundle By Name(w327) -> ("Repetitions"=w330:u16)
                        n309 = Select(t=i8 1, s=w326, f=w330) -> (s? t:f=w329:u16)
                        n310 = for {
                          N: w329 -> [w359]
                          tunnel: w322 -> [w351]
                          shift-right: [w364] -> _
                          shift-left: u16[][] [] -> [w365]
                          tunnel: w325 -> [w346]
                          tunnel: w324 -> [w345]
                          tunnel: w323 -> [w344]
                          i -> [w360]
                          stop <- w363 continue-if-true
                          w339 = u16 0 items=["Pixel", "Wavelength", "Energy"] ("Spectrum Axis")
                          w342 = u16 2 items=["Pixel", "Wavelength", "Energy"] ("Spectrum Axis")
                          n311 = Number To Decimal String(number=w359) -> (decimal integer string=w358:string)  [unwired: 1 in]
                          n312 = Increment(x=w360) -> (x+1=w356:i32)
                          n313 = call "Symphony Acquire Spectrum.vi"("Acquire"=w345, "Running"=w346, "Error In"=w344, "ShutterOpen"=TRUE, "JYCCDLib.IJYCCDReqd"=w351) -> ("Acq Time(ms)"=w343:u32, "Raw Data"=w349:i32[][])  [unwired: 5 in]
                          n314 = Number To Decimal String(number=w356) -> (decimal integer string=w357:string)  [unwired: 1 in]
                          n315 = local write "CCD Timing"(w343) -> ()
                          n316 = Index Array(array=w349, index (row)=0) -> (element=w347:i32[])  [unwired: 1 in]
                          n317 = Concatenate Strings(w357, "/" ("string"), w358) -> (w362:string)
                          n318 = local write "CCD Current Rep."(w362) -> ()
                          n319 = Build Array (concatenate)(w347, w365) -> (w364:i32[][])
                          n320 = local read "Wavelengths (nm)"() -> (w337:dbl[])
                          n321 = local read "Spectrum Axis"() -> (w340:u16)
                          n322 = local read "CCD Area"() -> (w336:T2)
                          n323 = call "Symphony Average Spectra.vi"("Repetitions"=w356, "Raw Spectra"=w364) -> ("Raw Spectrum"=w335:dbl[])
                          n324 = Not Equal?(x=w339, y=w340) -> (x != y?=w338:bool)
                          n325 = Equal?(x=w340, y=w342) -> (x = y?=w341:bool)
                          n326 = call "Spectrum Merge Pixels v10.5.0.vi"("CCD Area Format"=w336, "Raw Spectrum"=w335) -> ("Spectrum-Array"=w333:dbl[][])  [unwired: 1 out]
                          n327 = call "Spectrum Merge Wavelengths v10.5.0.vi"("Wavelengths (nm)"=w337, "Raw Spectrum"=w335) -> ("Spectrum-Array"=w332:dbl[][])  [unwired: 1 out]
                          n328 = local read "Spectrum Noise"() -> (w355:i64)
                          n329 = case shown="False" w338 {
                            tunnel: [w366 w367] -> w334
                            tunnel: w332 -> [_ w367]
                            tunnel: w333 -> [w366 _]
                            frame False {
                            }
                            frame True {
                            }
                          }
                          n330 = call "Spectrum Noise Subtraction v10.5.0.vi"("Spectrum Noise"=w355, "Spectrum-Array In"=w334) -> ("Spectrum-Array Out"=w354:dbl[][], "Spectrum-Cluster"=w352:T20)
                          n331 = local write "Spectrum Raw PX"(w333) -> ()
                          n332 = local write "Spectrum Raw WL"(w332) -> ()
                          n333 = case shown="True" w341 {
                            tunnel: w354 -> [_ w370]
                            tunnel: [w368 w369] -> w353
                            tunnel: w352 -> [w368 _]
                            frame False {
                            }
                            frame True {
                              n334 = call "Spectrum Jacobian Transformation v10.5.0.vi"("Spectrum-Array In"=w370) -> ("Spectrum-Cluster"=w369:T20)  [unwired: 1 in, 1 out]
                            }
                          }
                          n335 = local read "CCD Acquire"() -> (w363:bool)
                          n336 = local write "Spectrum"(w353) -> ()
                        }
                      }
                      frame True {
                        n337 = call "Symphony Acquire Image.vi"("Acquire"=w375, "Running"=w376, "Error In"=w377, "ShutterOpen"=TRUE, "JYCCDLib.IJYCCDReqd"=w378) -> ("Acq Time(ms)"=w371:u32, "Raw Data"=w374:i32[][][])  [unwired: 5 in]
                        n338 = local write "CCD Timing"(w371) -> ()
                        n339 = Index Array(array=w374, index (dim 0)=0 ("index (row)")) -> (element=w372:i32[][])  [unwired: 2 in]
                        n340 = local write "Image Raw"(w372) -> ()
                        n341 = local write "Image"(w372) -> ()
                      }
                    }
                  }
                  frame #1 {
                    n342 = local write "CCD Acquire"(FALSE ("Blinkend")) -> ()
                    n343 = local write "CCD Current Rep."("0/0" ("CCD3000 Current Rep.")) -> ()
                    n344 = local read "Graph Supersize Ref"() -> (w380:refnum<vi>)
                    n345 = Equal?(x=w380, y=refnum<k0> refnum) -> (x = y?=w382:bool)
                    n346 = local read "Spectrum Autosave"() -> (w385:bool)
                    n347 = case shown="False" w382 {
                      tunnel: w380 -> [w386 _]
                      frame False {
                        n348 = property class="VI"(reference=w386) -> ("FP.State"=w389:T18)  [unwired: 1 in, 2 out]
                        n349 = Greater Or Equal?(x=w389, y=T18."Hidden") -> (x >= y?=w387:bool)
                        n350 = case shown="True" w387 {
                          frame False {
                          }
                          frame True {
                            n351 = property on="Update Supersize" class="Bool (strict)"("Val(Sgnl)"=TRUE ("Value (Signaling)")) -> ()  [unwired: 2 in, 2 out]
                          }
                        }
                      }
                      frame True {
                      }
                    }
                    n352 = case shown="True" w385 {
                      frame False {
                      }
                      frame True {
                        n353 = property on="Spectrum Save" class="Bool (strict)"("Val(Sgnl)"=TRUE ("Value (Signaling)")) -> ()  [unwired: 2 in, 2 out]
                      }
                    }
                  }
                }
              }
            }
          }
          event "Image Mode": Value Change {
            # "For Symphony (II), ADC0 is\n20 kHz and ADC1 is 1 MHz.\nThis couples the selected  ADC\nto the imaging mode selection."
            n354 = event-data() -> ("NewVal"=w395:bool)  [unwired: 1 in, 4 out]
            n355 = Select(t=i8 1, s=w395, f=i8 0) -> (s? t:f=w394:i8)
            n356 = property on="CCD ADC" class="Ring (strict)"("Val(Sgnl)"=w394) -> ()  [unwired: 2 in, 2 out]
          }
          event "CCD Preview": Value Change {
            n357 = event-data() -> ("NewVal"=w396:bool)  [unwired: 1 in, 4 out]
            n358 = case shown="False" w396 {
              frame False {
              }
              frame True {
                n359 = property on="CCD Acquire" class="Bool (strict)"("Val(Sgnl)"=TRUE ("Wert (signalisierend)")) -> ()  [unwired: 2 in, 2 out]
              }
            }
          }
          event "ITC Connect": Value Change {
            n360 = event-data() -> ("NewVal"=w398:bool)  [unwired: 1 in, 4 out]
            n361 = stacked-sequence {
              tunnel: w398 -> [_ w400 _]
              frame #0 {
                n362 = property on="ITC Running" class="Bool (strict)"("Blinking"=TRUE ("Blinkend")) -> ()  [unwired: 2 in, 2 out]
              }
              frame #1 {
                n363 = case shown="False" w400 {
                  selector: w400 -> [w405 _]
                  tunnel: [w405 w412] -> w402
                  frame False {
                    # "disconnect"
                    n364 = control-ref of="ITC Running"() -> (w406:refnum<vi>)
                    n365 = property class="Bool (strict)"(reference=w406, "Blinking"=w405, "Value"=w405) -> ()  [unwired: 1 in, 2 out]
                  }
                  frame True {
                    # "connect"
                    n366 = local read "ITC Selector"() -> (w413:u16)
                    n367 = call "ITC503 Connect.vi"("ITC Selector"=w413) -> ("ITC Setup"=w411:T11, "Connected"=w412:bool)
                    n368 = local write "ITC Setup"(w411) -> ()
                    n369 = call "ITC503 Get Values.vi"("ITC Setup"=w411) -> ("ITC503 Current Values"=w410:T3)  [unwired: 1 in, 1 out]
                    n370 = Unbundle By Name(w410) -> ("ITC503 Setpoint"=w407:dbl)
                    n371 = Bundle By Name(cluster=T4 {"ITC503 Set Setpoint"=0.0, "ITC503 Set Auto Heater"=TRUE, "ITC503 Set Auto PID"=TRUE, "P"=0.0, "I"=0.0, "D"=0.0} ("ITC503 Settings"), "ITC503 Set Setpoint"=w407) -> (w408:T4)
                    n372 = local write "ITC Settings"(w408) -> ()
                  }
                }
                n373 = case shown="False" w402 {
                  tunnel: [T15."Disabled and Grayed Out" ("Deaktiviert") T15."Enabled" ("Deaktiviert")] -> w401
                  frame False {
                  }
                  frame True {
                  }
                }
                n374 = local write "ITC Status"(w402) -> ()
                n375 = local write "ITC Connect"(w402) -> ()
                n376 = property on="ITC Configure" class="Bool (strict)"("DisabledEnum"=w401) -> ()  [unwired: 2 in, 2 out]
              }
              frame #2 {
                n377 = property on="ITC Running" class="Bool (strict)"("Blinking"=FALSE ("Blinkend")) -> ()  [unwired: 2 in, 2 out]
                n378 = property on="ITC Read" class="Bool (strict)"("Val(Sgnl)"=TRUE ("Wert (signalisierend)")) -> ()  [unwired: 2 in, 2 out]
              }
            }
          }
          event "ITC Read": Value Change {
            n379 = event-data() -> ("Time"=w417:u32, "NewVal"=w420:bool)  [unwired: 1 in, 3 out]
            n380 = local read "ITC Status"() -> (w419:bool)
            n381 = And(x=w419, y=w420) -> (x .and. y?=w418:bool)
            n382 = case shown="True" w418 {
              tunnel: w417 -> [_ w424]
              tunnel: [u32 0 w423] -> w416
              frame False {
                n383 = property on="ITC Running" class="Bool (strict)"("BoolText.Text"="" ("Boolescher Text.Text")) -> ()  [unwired: 2 in, 2 out]
              }
              frame True {
                n384 = stacked-sequence {
                  seq-local: [_ w430 _ _] -> [_ _ w451 _]
                  seq-local: [w425 _ _ _] -> [_ _ _ w459]
                  tunnel: w424 -> [_ w431 _ _]
                  tunnel: [_ _ _ w460] -> w423
                  frame #0 {
                    n385 = Tick Count (ms)() -> (millisecond timer value=w425:u32)
                  }
                  frame #1 {
                    n386 = local read "ITC Setup"() -> (w436:T11)
                    n387 = local read "ITC Gradient Time"() -> (w435:i64)
                    n388 = call "ITC503 Get Values.vi"("ITC Setup"=w436) -> ("ITC503 Current Values"=w430:T3)  [unwired: 1 in, 1 out]
                    n389 = local read "ITC Temp Storage"() -> (w429:dbl)
                    n390 = Unbundle By Name(w430) -> ("ITC503 Temperature"=w428:dbl)
                    n391 = Subtract(x=w431, y=w435) -> (x-y=w434:i64)
                    n392 = Divide(x=w434, y=i64 1000) -> (x/y=w432:dbl)
                    n393 = Equal To 0?(x=w428) -> (x = 0?=w427:bool)
                    n394 = case shown="False" w427 {
                      tunnel: w432 -> [w442 _]
                      tunnel: w430 -> [w441 _]
                      tunnel: w429 -> [w440 _]
                      tunnel: w428 -> [w438 _]
                      frame False {
                        n395 = Subtract(x=w438, y=w440) -> (x-y=w439:dbl)
                        n396 = Divide(x=w439, y=w442) -> (x/y=w443:dbl)
                        n397 = Bundle By Name(cluster=w441, "ITC503 Gradient"=w443) -> (w437:T3)
                        n398 = local write "ITC Current Values"(w437) -> ()
                        n399 = global write "Global Variables.vi" "Global ITC Values"(w437) -> ()
                      }
                      frame True {
                      }
                    }
                    n400 = Not(x=w427) -> (.not. x?=w426:bool)
                    n401 = local write "ITC Status"(w426) -> ()
                  }
                  frame #2 {
                    n402 = Unbundle By Name(w451) -> ("ITC503 Temperature"=w446:dbl, "ITC503 Setpoint"=w452:dbl)
                    n403 = Subtract(x=w446, y=w452) -> (x-y=w453:dbl)
                    n404 = Number To Fractional String(number=w446, precision (6)=i16 2 ("Genauigkeit (6)")) -> (F-format string=w449:string)  [unwired: 2 in]
                    n405 = local write "ITC Temp Storage"(w446) -> ()
                    n406 = Absolute Value(x=w453) -> (abs(x)=w454:dbl)
                    n407 = String Subset(string=w449, length (rest)=5 ("Länge (Rest)")) -> (substring=w447:string)  [unwired: 1 in]
                    n408 = Less?(x=w454, y=2.0) -> (x < y?=w445:bool)
                    n409 = case shown="True" w445 {
                      tunnel: [u32 16711680 u32 0] -> w444
                      frame False {
                      }
                      frame True {
                      }
                    }
                    n410 = property on="ITC Running" class="Bool (strict)"("Value"=w445, "BoolText.Text"=w447, "BoolText.TextColor"=w444) -> ()  [unwired: 2 in, 2 out]
                  }
                  frame #3 {
                    n411 = Tick Count (ms)() -> (millisecond timer value=w458:u32)
                    n412 = local write "ITC Gradient Time"(w458) -> ()
                    n413 = Subtract(x=w458, y=w459) -> (x-y=w460:u32)
                  }
                }
              }
            }
            n414 = local write "ITC Timing"(w416) -> ()
          }
          event "ITC Configure": Value Change {
            n415 = event-data() -> ("NewVal"=w461:bool)  [unwired: 1 in, 4 out]
            n416 = stacked-sequence {
              tunnel: w461 -> [_ w463 _]
              frame #0 {
                n417 = property on="ITC Running" class="Bool (strict)"("Blinking"=TRUE ("Blinkend")) -> ()  [unwired: 2 in, 2 out]
              }
              frame #1 {
                n418 = local read "ITC Status"() -> (w465:bool)
                n419 = And(x=w465, y=w463) -> (x .and. y?=w464:bool)
                n420 = case shown="True" w464 {
                  frame False {
                  }
                  frame True {
                    n421 = local read "ITC Settings"() -> (w466:T4)
                    n422 = local read "ITC Setup"() -> (w467:T11)
                    n423 = call "ITC503 Set Values.vi"("Set Channel"=i16 1, "ITC503 Settings"=w466, "ITC Setup"=w467) -> ()  [unwired: 2 in]
                  }
                }
              }
              frame #2 {
                w470 = FALSE ("Blinkend")
                n424 = property on="ITC Running" class="Bool (strict)"("Blinking"=w470) -> ()  [unwired: 2 in, 2 out]
                n425 = local write "ITC Configure"(w470) -> ()
                n426 = property on="ITC Read" class="Bool (strict)"("Val(Sgnl)"=TRUE ("Wert (signalisierend)")) -> ()  [unwired: 2 in, 2 out]
              }
            }
          }
          event "Drive Connect": Value Change {
            n427 = event-data() -> ("NewVal"=w471:bool)  [unwired: 1 in, 4 out]
            n428 = stacked-sequence {
              tunnel: w471 -> [_ w475 _ _]
              frame #0 {
                n429 = property on="Drive Running" class="Bool (strict)"("Blinking"=TRUE ("Blinkend")) -> ()  [unwired: 2 in, 2 out]
              }
              frame #1 {
                n430 = local read "Drive Connection"() -> (w476:refnum<visa-resource-name>)
                n431 = local read "Drive Calibration"() -> (w473:path)
                n432 = case shown="True" w475 {
                  tunnel: w476 -> [w481 w484]
                  tunnel: [TRUE ("Success") w483] -> w474
                  tunnel: w473 -> [_ w482]
                  frame False {
                    n433 = call "NPC3SG Close.vi"("Drive Visa Name"=w481) -> ()  [unwired: 4 in]
                  }
                  frame True {
                    n434 = call "NPC3SG Connect v10.6.2.vi"("Calibration File"=w482, "Drive Port"=w484) -> ("Success"=w483:bool)  [unwired: 1 in, 1 out]
                  }
                }
                n435 = Not(x=w475) -> (.not. x?=w478:bool)
                n436 = Exclusive Or(1:w478, 2:w474) -> (0:w479:bool)
                n437 = local write "Drive Connect"(w479) -> ()
                n438 = local write "Drive Status"(w479) -> ()
                n439 = case shown="False" w479 {
                  tunnel: [T15."Disabled and Grayed Out" ("Deaktiviert") T15."Enabled" ("Deaktiviert")] -> w477
                  frame False {
                  }
                  frame True {
                  }
                }
                n440 = property on="Drive Live Controls" class="Clust (strict)"("DisabledEnum"=w477) -> ()  [unwired: 2 in, 2 out]
                n441 = property on="Drive GoTo" class="Bool (strict)"("DisabledEnum"=w477) -> ()  [unwired: 2 in, 2 out]
              }
              frame #2 {
                # "prepare mirroring values to target controls"
                n442 = local write "Drive Copy Target"(TRUE ("Copy Drive Target")) -> ()
              }
              frame #3 {
                n443 = property on="Drive Running" class="Bool (strict)"("Blinking"=FALSE ("Blinkend")) -> ()  [unwired: 2 in, 2 out]
                n444 = property on="Drive Read" class="Bool (strict)"("Val(Sgnl)"=TRUE ("Wert (signalisierend)")) -> ()  [unwired: 2 in, 2 out]
              }
            }
          }
          event "Drive Read": Value Change {
            n445 = event-data() -> ("NewVal"=w493:bool)  [unwired: 1 in, 4 out]
            n446 = local read "Drive Status"() -> (w492:bool)
            n447 = And(x=w492, y=w493) -> (x .and. y?=w491:bool)
            n448 = case shown="True" w491 {
              tunnel: [u32 0 w495] -> w490
              frame False {
              }
              frame True {
                n449 = stacked-sequence {
                  seq-local: [w496 _ _ _] -> [_ _ _ w503]
                  tunnel: [_ _ _ w502] -> w495
                  frame #0 {
                    n450 = Tick Count (ms)() -> (millisecond timer value=w496:u32)
                  }
                  frame #1 {
                    n451 = local read "Drive Calibration"() -> (w497:path)
                    n452 = local read "Drive Connection"() -> (w499:refnum<visa-resource-name>)
                    n453 = call "NPC3SG Get Positions v10.6.2.vi"("Drive Visa Name"=w499, "Calibration File"=w497) -> ("Drive Current Values"=w498:T1)  [unwired: 5 in]
                    n454 = local write "Drive Live Current Values"(w498) -> ()
                    n455 = local write "Drive Current Values"(w498) -> ()
                    n456 = global write "Global Variables.vi" "Global Piezo Position"(w498) -> ()
                  }
                  frame #2 {
                    n457 = local read "Drive Copy Target"() -> (w500:bool)
                    n458 = case shown="True" w500 {
                      frame False {
                      }
                      frame True {
                        n459 = property on="Drive Copy Target" class="Bool (strict)"("Val(Sgnl)"=TRUE ("Value (Signaling)")) -> ()  [unwired: 2 in, 2 out]
                      }
                    }
                  }
                  frame #3 {
                    n460 = Tick Count (ms)() -> (millisecond timer value=w504:u32)
                    n461 = Subtract(x=w504, y=w503) -> (x-y=w502:u32)
                  }
                }
              }
            }
            "Drive Timing" <- w490
          }
          event "Drive GoTo": Value Change {
            n462 = event-data() -> ("NewVal"=w505:bool)  [unwired: 1 in, 4 out]
            n463 = stacked-sequence {
              tunnel: w505 -> [_ w507 _]
              frame #0 {
                n464 = property on="Drive Running" class="Bool (strict)"("Blinking"=TRUE ("Blinkend")) -> ()  [unwired: 2 in, 2 out]
              }
              frame #1 {
                n465 = local read "Drive Status"() -> (w509:bool)
                n466 = And(x=w509, y=w507) -> (x .and. y?=w508:bool)
                n467 = case shown="True" w508 {
                  frame False {
                  }
                  frame True {
                    n468 = local read "Drive New Positions"() -> (w512:T6)
                    n469 = local read "Drive Calibration"() -> (w510:path)
                    n470 = local read "Drive Connection"() -> (w511:refnum<visa-resource-name>)
                    n471 = control-ref of="Drive Running"() -> (w513:refnum<vi>)
                    n472 = call "NPC3SG Move Absolute v10.6.2.vi"("Running"=w513, "Calibration File"=w510, "Drive New Abs. Positions"=w512, "Drive Visa Name"=w511) -> ()  [unwired: 1 in]
                  }
                }
              }
              frame #2 {
                w515 = FALSE ("Blinkend")
                n473 = local write "Drive GoTo"(w515) -> ()
                n474 = property on="Drive Running" class="Bool (strict)"("Blinking"=w515) -> ()  [unwired: 2 in, 2 out]
                n475 = property on="Drive Read" class="Bool (strict)"("Val(Sgnl)"=TRUE ("Wert (signalisierend)")) -> ()  [unwired: 2 in, 2 out]
              }
            }
          }
          event Value Change {
            n476 = event-data() -> ("NewVal"=w517:bool)  [unwired: 1 in, 4 out]
            n477 = local read "Drive Status"() -> (w518:bool)
            n478 = And(x=w518, y=w517) -> (x .and. y?=w516:bool)
            n479 = case shown="True" w516 {
              frame False {
              }
              frame True {
                n480 = stacked-sequence {
                  seq-local: [w519 _ _] -> [_ _ _]
                  frame #0 {
                    # "Move and Read"
                    n481 = flat-sequence {
                      tunnel: [w527] -> w522
                      tunnel: [w525] -> w521
                      tunnel: w522 -> [w529]
                      tunnel: w521 -> [w530]
                      tunnel: [w528] -> w520
                      tunnel: w520 -> [w535]
                      tunnel: [w535] -> w519
                      frame #0 {
                        n482 = local read "Drive Live Controls"() -> (w525:T7)
                        n483 = local read "Drive Connection"() -> (w524:refnum<visa-resource-name>)
                        n484 = local read "Drive Calibration"() -> (w523:path)
                        n485 = control-ref of="Drive Running"() -> (w526:refnum<vi>)
                        n486 = call "NPC3SG Live Control v10.6.2.vi"("Running"=w526, "Calibration File"=w523, "Drive Live Controls"=w525, "Drive Visa Name"=w524) -> ("Reset Switches"=w527:bool)
                      }
                      frame #1 {
                        n487 = case shown="True" w529 {
                          tunnel: w530 -> [w531 w534]
                          tunnel: [w531 w533] -> w528
                          frame False {
                          }
                          frame True {
                            w532 = FALSE ("Move Out")
                            n488 = Bundle By Name(cluster=w534, "Move Home"=w532, "Move Down"=w532, "Move Up"=w532, "Move Left"=w532, "Move Right"=w532, "Move Out"=w532, "Move In"=w532) -> (w533:T7)
                          }
                        }
                      }
                      frame #2 {
                        n489 = local write "Drive Live Controls"(w535) -> ()
                      }
                    }
                  }
                  frame #1 {
                    n490 = local write "Drive Copy Target"(TRUE ("Copy Drive Target")) -> ()
                  }
                  frame #2 {
                    n491 = property on="Drive Read" class="Bool (strict)"("Val(Sgnl)"=TRUE ("Wert (signalisierend)")) -> ()  [unwired: 2 in, 2 out]
                  }
                }
              }
            }
          }
          event "Drive Copy Target": Value Change {
            # "this event is triggered after drive readout\nit should usually not be triggered directly by signaling"
            n492 = event-data() -> ("NewVal"=w538:bool)  [unwired: 1 in, 4 out]
            n493 = case shown="True" w538 {
              frame False {
              }
              frame True {
                n494 = stacked-sequence {
                  frame #0 {
                    n495 = local read "Drive Current Values"() -> (w539:T1)
                    n496 = local write "Drive New Positions"(w539) -> ()
                  }
                  frame #1 {
                    n497 = local write "Drive Copy Target"(FALSE ("Copy Drive Target")) -> ()
                  }
                }
              }
            }
          }
          event "Wavelength Recalculate": Value Change {
            n498 = event-data() -> ("NewVal"=w541:bool)  [unwired: 1 in, 4 out]
            n499 = case shown="False" w541 {
              frame False {
              }
              frame True {
                n500 = local read "Mono Current Values"() -> (w544:T9)
                n501 = local read "CCD Area"() -> (w542:T2)
                n502 = call "iHR550 Convert Axis v10.5.0.vi"("CCD Area Format"=w542, "iHR Current Values"=w544) -> ("Wavelengths (nm)"=w543:dbl[])
                n503 = local write "Wavelengths (nm)"(w543) -> ()
                n504 = global write "Global Variables.vi" "Global Wavelengths (nm)"(w543) -> ()
              }
            }
          }
          event Value Change {
            n505 = event-data() -> ("NewVal"=w546:dbl)  [unwired: 1 in, 4 out]
            n506 = local read "JYCCDLib.IJYCCDReqd"() -> (w545:refnum<k7>)
            n507 = call "Symphony Set Integration Time.vi"("JYCCDLib.IJYCCDReqd"=w545, "Integration (s)"=w546) -> ()  [unwired: 13 in, 1 out]
          }
          event "Spectrum Axis": Value Change {
            w559 = u16 2 items=["Pixel", "Wavelength", "Energy"] ("Spectrum Axis")
            w561 = u16 0 items=["Pixel", "Wavelength", "Energy"] ("Spectrum Axis")
            n508 = event-data() -> ("NewVal"=w557:u16)  [unwired: 1 in, 4 out]
            n509 = Equal?(x=w557, y=w561) -> (x = y?=w560:bool)
            n510 = case shown="True" w560 {
              tunnel: [w579 w581] -> w558
              tunnel: [w578 w580] -> w553
              tunnel: "Pixel" ("X Scale.Name Label.Text") -> [_ w580]
              tunnel: "Wavelength (nm)" ("X Scale.Name Label.Text") -> [w578 _]
              frame False {
                n511 = local read "Spectrum Raw WL"() -> (w579:dbl[][])
              }
              frame True {
                n512 = local read "Spectrum Raw PX"() -> (w581:dbl[][])
              }
            }
            n513 = local read "Spectrum Noise"() -> (w548:i64)
            n514 = Equal?(x=w557, y=w559) -> (x = y?=w556:bool)
            n515 = call "Spectrum Noise Subtraction v10.5.0.vi"("Spectrum Noise"=w548, "Spectrum-Array In"=w558) -> ("Spectrum-Array Out"=w555:dbl[][], "Spectrum-Cluster"=w547:T20)
            n516 = case shown="True" w556 {
              tunnel: w555 -> [_ w569]
              tunnel: [w563 w568] -> w554
              tunnel: w547 -> [w563 w567]
              tunnel: w553 -> [w562 w564]
              tunnel: [w562 w566] -> w550
              tunnel: "Energy (eV)" ("X Scale.Name Label.Text") -> [_ w565]
              tunnel: w548 -> [_ w570]
              frame False {
              }
              frame True {
                # "Jacobian Transformation requires noise subtraction"
                n517 = Greater Than 0?(x=w570) -> (x > 0?=w571:bool)
                n518 = case shown="False" w571 {
                  tunnel: w569 -> [_ w577]
                  tunnel: [w573 w576] -> w568
                  tunnel: w567 -> [w573 _]
                  tunnel: [w572 w575] -> w566
                  tunnel: w565 -> [_ w575]
                  tunnel: w564 -> [w572 _]
                  frame False {
                    w574 = u16 1 items=["Pixel", "Wavelength", "Energy"] ("Spectrum Axis")
                    n519 = call "Display Message to User"() -> ()  [unwired: 10 in, 2 out]
                    n520 = local write "Spectrum Axis"(w574) -> ()
                  }
                  frame True {
                    n521 = call "Spectrum Jacobian Transformation v10.5.0.vi"("Spectrum-Array In"=w577) -> ("Spectrum-Cluster"=w576:T20)  [unwired: 1 in, 1 out]
                  }
                }
              }
            }
            n522 = local write "Spectrum"(w554) -> ()
            n523 = property on="Spectrum" class="XYGraph (strict)"("XScale.NameLbl.Text"=w550) -> ()  [unwired: 2 in, 2 out]
          }
          event "Spectrum Noise": Value Change {
            n524 = event-data() -> ("NewVal"=w584:i64)  [unwired: 1 in, 4 out]
            n525 = Greater Than 0?(x=w584) -> (x > 0?=w583:bool)
            n526 = case shown="False" w583 {
              tunnel: [w585 w586] -> w582
              frame False {
                w585 = u16 1 items=["Pixel", "Wavelength", "Energy"] ("Spectrum Axis")
                # "Disable Jacobian Transformation"
              }
              frame True {
                n527 = local read "Spectrum Axis"() -> (w586:u16)
              }
            }
            n528 = property on="Spectrum Axis" class="Ring (strict)"("Val(Sgnl)"=w582) -> ()  [unwired: 2 in, 2 out]
          }
          event "Spectrum Save": Value Change {
            n529 = event-data() -> ("NewVal"=w587:bool)  [unwired: 1 in, 4 out]
            n530 = stacked-sequence {
              tunnel: w587 -> [w588 _]
              frame #0 {
                n531 = case shown="True" w588 {
                  frame False {
                  }
                  frame True {
                    n532 = local read "Mono Current Values"() -> (w591:T9)
                    n533 = local read "Drive Current Values"() -> (w589:T1)
                    n534 = local read "ITC Current Values"() -> (w592:T3)
                    n535 = local read "Spectrum Settings"() -> (w590:T5)
                    n536 = local read "CCD Temperature"() -> (w597:dbl)
                    n537 = local read "CCD Area"() -> (w594:T2)
                    n538 = local read "CCD ADC"() -> (w596:u16)
                    n539 = local read "CCD Gain"() -> (w595:u16)
                    n540 = local read "Image Mode"() -> (w603:bool)
                    n541 = call "Export_fileName v10.6.0.vi"("ITC503 Current Values"=w592, "iHR Current Values"=w591, "Spectra Settings"=w590, "Drive Current Values"=w589) -> ("Filename"=w593:string)  [unwired: 1 in]
                    n542 = case shown="True" w603 {
                      tunnel: [w604 w608] -> w601
                      tunnel: ["Spectrum" ("Export Type") "Image" ("Export Type")] -> w600
                      tunnel: [w605 w612] -> w598
                      tunnel: w594 -> [_ w607]
                      tunnel: w593 -> [w604 w610]
                      frame False {
                        n543 = local read "Spectrum Raw WL"() -> (w605:dbl[][])
                      }
                      frame True {
                        n544 = local read "Image Raw"() -> (w611:i32[][])
                        n545 = Concatenate Strings(w610, "_img" ("string")) -> (w608:string)
                        n546 = call "Image Merge Axes v10.5.1.vi"("Image In"=w611, "CCD Area Format"=w607) -> ("Image Out"=w612:dbl[][])  [unwired: 13 in]
                      }
                    }
                    n547 = local read "Spectrum Autosave"() -> (w599:bool)
                    n548 = local read "Auto Folder"() -> (w602:path)
                    n549 = call "Export_2DtoTxt v10.6.3.vi"("ITC503 Current Values"=w592, "iHR Current Values"=w591, "CCD Temperature"=w597, "CCD Area"=w594, "CCD ADC"=w596, "CCD Gain"=w595, "Auto?"=w599, "Export Type"=w600, "Spectra Settings"=w590, "Filename"=w601, "Data (2D)"=w598, "Auto Folder"=w602) -> ()  [unwired: 7 in, 1 out]
                  }
                }
              }
              frame #1 {
                n550 = local write "Spectrum Save"(FALSE ("Spectrum Save")) -> ()
              }
            }
          }
          event "Spectrum Load": Value Change {
            n551 = event-data() -> ("NewVal"=w615:bool)  [unwired: 1 in, 4 out]
            n552 = case shown="True" w615 {
              frame False {
              }
              frame True {
                n553 = stacked-sequence {
                  seq-local: [w616 _ _] -> [_ w619 _]
                  frame #0 {
                    n554 = call "Load Spectrum.vi"() -> ("Intensity"=w616:dbl[], "Wavelength"=w618:dbl[])  [unwired: 3 in, 1 out]
                    n555 = Build Array(w618, w616) -> (w617:dbl[][])
                    n556 = local write "Spectrum Raw WL"(w617) -> ()
                  }
                  frame #1 {
                    n557 = call <vilib>:"Median.vi"("X"=w619) -> ("median"=w621:dbl)  [unwired: 1 out]
                    n558 = To Long Integer(number=w621) -> (32bit integer=w620:i32)
                    n559 = property on="Spectrum Noise" class="DigNum (strict)"("Val(Sgnl)"=w620) -> ()  [unwired: 2 in, 2 out]
                  }
                  frame #2 {
                    n560 = local write "Spectrum Load"(FALSE ("Spectrum Load")) -> ()
                  }
                }
              }
            }
          }
          event "Spectrum Autosave": Value Change {
            n561 = event-data() -> ("NewVal"=w624:bool)  [unwired: 1 in, 4 out]
            n562 = case shown="False" w624 {
              tunnel: [path "" w630] -> w623
              frame False {
              }
              frame True {
                n563 = call "File Dialog"("prompt"="Choose Save Folder") -> ("selected path"=w632:path, "cancelled"=w626:bool, "error out"=w628:errorcluster)  [unwired: 11 in, 1 out]
                n564 = call <vilib>:"Simple Error Handler.vi"("error in (no error)"=w628) -> ("error?"=w627:bool)  [unwired: 4 in, 4 out]
                n565 = Or(x=w626, y=w627) -> (x .or. y?=w629:bool)
                n566 = case shown="True" w629 {
                  tunnel: w632 -> [w633 _]
                  tunnel: [w633 path ""] -> w630
                  frame False {
                  }
                  frame True {
                    n567 = local write "Spectrum Autosave"(FALSE ("Spectrum Autosave")) -> ()
                  }
                }
              }
            }
            n568 = local write "Auto Folder"(w623) -> ()
          }
          event "Graph Maximize": Value Change {
            n569 = event-data() -> ("NewVal"=w636:bool)  [unwired: 1 in, 4 out]
            n570 = case shown="True" w636 {
              frame False {
              }
              frame True {
                n571 = local read "Image Mode"() -> (w652:bool)
                n572 = local write "Graph Maximize"(FALSE ("Graph Maximize")) -> ()
                n573 = vi-ref "Graph Supersize v10.6.2.vi"() -> (w651:refnum<vi>)
                n574 = invoke class="VI" method="Ctrl Val.Set"(reference=w651, "Control Name"="Image Mode", "Value"=w652) -> (reference out=w642:refnum<vi>, error out=w641:errorcluster)  [unwired: 2 in, 3 out]
                n575 = invoke class="VI" method="Ctrl Val.Set"(reference=w642, error in=w641, "Control Name"="AutoClose", "Value"=TRUE ("Activate?")) -> (reference out=w639:refnum<vi>, error out=w640:errorcluster)  [unwired: 1 in, 3 out]
                n576 = invoke on="Invoke Node" class="VI" method="FP.Open"(reference=w639, error in=w640, "Activate"=TRUE ("Activate?")) -> (reference out=w648:refnum<vi>, error out=w649:errorcluster)  [unwired: 2 in, 3 out]
                n577 = invoke on="Invoke Node" class="VI" method="Run VI"(reference=w648, error in=w649, "Wait until done"=FALSE ("Wait Until Done"), "Auto Dispose Ref"=TRUE ("Auto Dispose Reference")) -> (reference out=w643:refnum<vi>)  [unwired: 1 in, 4 out]
                n578 = local write "Graph Supersize Ref"(w643) -> ()
              }
            }
          }
          event "Update Supersize": Value Change {
            n579 = event-data() -> ("NewVal"=w653:bool)  [unwired: 1 in, 4 out]
            n580 = case shown="True" w653 {
              frame False {
              }
              frame True {
                n581 = local read "Graph Supersize Ref"() -> (w658:refnum<vi>)
                n582 = local read "Image Mode"() -> (w655:bool)
                n583 = invoke class="VI" method="Ctrl Val.Set"(reference=w658, "Control Name"="Image Mode", "Value"=w655) -> (reference out=w657:refnum<vi>, error out=w656:errorcluster)  [unwired: 2 in, 3 out]
                n584 = case shown="False" w655 {
                  tunnel: w657 -> [w664 w670]
                  tunnel: w656 -> [w663 w667]
                  frame False {
                    n585 = local read "Spectrum"() -> (w665:cluster{dbl[], dbl[]}[])
                    n586 = invoke class="VI" method="Ctrl Val.Set"(reference=w664, error in=w663, "Control Name"="Spectrum", "Value"=w665) -> (reference out=w662:refnum<vi>, error out=w661:errorcluster)  [unwired: 1 in, 3 out]
                    n587 = property on="Spectrum" class="XYGraph (strict)"() -> ("XScale.NameLbl.Text"=w659:string)  [unwired: 2 in, 2 out]
                    n588 = invoke class="VI" method="Ctrl Val.Set"(reference=w662, error in=w661, "Control Name"="SpectrumAxis", "Value"=w659) -> ()  [unwired: 1 in, 5 out]
                  }
                  frame True {
                    n589 = local read "Image"() -> (w668:dbl[][])
                    n590 = invoke class="VI" method="Ctrl Val.Set"(reference=w670, error in=w667, "Control Name"="Image", "Value"=w668) -> ()  [unwired: 1 in, 5 out]
                  }
                }
              }
            }
          }
          event "Mapping Start": Value Change {
            n591 = event-data() -> ("NewVal"=w671:bool)  [unwired: 1 in, 4 out]
            n592 = case shown="True" w671 {
              frame False {
              }
              frame True {
                n593 = stacked-sequence {
                  frame #0 {
                    # "Make sure we do not try mapping in the image mode."
                    n594 = flat-sequence {
                      frame #0 {
                        n595 = property on="Image Mode" class="Bool (strict)"("Val(Sgnl)"=FALSE ("Value (Signaling)")) -> ()  [unwired: 2 in, 2 out]
                      }
                      frame #1 {
                        n596 = property on="CCD Configure" class="Bool (strict)"("Val(Sgnl)"=TRUE ("Value (Signaling)")) -> ()  [unwired: 2 in, 2 out]
                      }
                    }
                  }
                  frame #1 {
                    n597 = local read "JYCCDLib.IJYCCDReqd"() -> (w713:refnum<k7>)
                    n598 = local read "Drive Current Values"() -> (w708:T1)
                    n599 = local read "ITC Current Values"() -> (w710:T3)
                    n600 = local read "Mono Current Values"() -> (w709:T9)
                    n601 = local read "CCD Temperature"() -> (w715:dbl)
                    n602 = vi-ref "Mapping v10.6.4.vi"() -> (w696:refnum<vi>)
                    n603 = local read "Wavelengths (nm)"() -> (w711:dbl[])
                    n604 = local read "Drive Status"() -> (w707:bool)
                    n605 = local read "Drive Connection"() -> (w712:refnum<visa-resource-name>)
                    n606 = local read "Spectrum Settings"() -> (w714:T5)
                    n607 = local read "CCD Status"() -> (w705:bool)
                    n608 = local read "Drive Calibration"() -> (w674:path)
                    n609 = local read "CCD ADC"() -> (w676:u16)
                    n610 = local read "CCD Area"() -> (w678:T2)
                    n611 = local read "CCD Gain"() -> (w677:u16)
                    n612 = local read "CCD Status"() -> (w689:bool)
                    n613 = Not(x=w707) -> (.not. x?=w706:bool)
                    n614 = Not(x=w705) -> (.not. x?=w704:bool)
                    n615 = Not(x=w689) -> (.not. x?=w688:bool)
                    n616 = Bundle By Name(cluster=T19 {"Drive Connection Port"="", "ITC503 Current Values"={"ITC503 Heater"=0.0, "ITC503 Temperature"=0.0, "ITC503 P"=0.0, "ITC503 I"=0.0, "ITC503 D"=0.0, "ITC503 Setpoint"=0.0, "ITC503 Gradient"=0.0, "ITC503 Heater Auto"=FALSE, "ITC503 PID Auto"=FALSE}, "Wavelengths (nm)"=[], "Drive Current Values"={"Drive X Position"=0.0, "Drive Y Position"=0.0, "Drive Z Position"=0.0}, "iHR Current Values"={"iHR 550 Front Entrance"=0.0, "iHR550 Side Exit"=0.0, "iHR550 Wavelength"=897.9988, "iHR550 Exit Mirror"=2, "iHR550 Grating"="1", "Grating Index"=1}, "Spectra Settings"={"Integration Time"=1.0, "Repetitions"=1, "Mapping Spectra"=TRUE}, "CCD3500 Temperature"=0.0, "Simulate Drive"=FALSE, "Simulate Spectra"=FALSE, "JYCCDLib.IJYCCDReqd"=refnum, "CCD Area"={"XStart"=1, "YStart"=1, "XStop"=2048, "YStop"=512, "XBin"=1, "YBin"=1}, "CCD Gain"=1, "CCD ADC"=0, "Drive Calibration"=path ""} ("Input Parameters"), "JYCCDLib.IJYCCDReqd"=w713, "Drive Connection Port"=w712, "ITC503 Current Values"=w710, "Wavelengths (nm)"=w711, "Drive Current Values"=w708, "iHR Current Values"=w709, "Spectra Settings"=w714, "CCD3500 Temperature"=w715, "Simulate Drive"=w706, "Simulate Spectra"=w704, "CCD Area"=w678, "CCD Gain"=w677, "CCD ADC"=w676, "Drive Calibration"=w674) -> (w697:T19)
                    n617 = invoke class="VI" method="Ctrl Val.Set"(reference=w696, "Control Name"="Simulate Spectra", "Value"=w688) -> (reference out=w695:refnum<vi>, error out=w690:errorcluster)  [unwired: 2 in, 3 out]
                    n618 = local read "Drive Status"() -> (w687:bool)
                    n619 = Not(x=w687) -> (.not. x?=w686:bool)
                    n620 = invoke class="VI" method="Ctrl Val.Set"(reference=w695, error in=w690, "Control Name"="Simulate Drive", "Value"=w686) -> (reference out=w694:refnum<vi>, error out=w691:errorcluster)  [unwired: 1 in, 3 out]
                    n621 = invoke class="VI" method="Ctrl Val.Set"(reference=w694, error in=w691, "Control Name"="Input Parameters", "Value"=w697) -> (reference out=w684:refnum<vi>, error out=w681:errorcluster)  [unwired: 1 in, 3 out]
                    n622 = property on="Measurement Running" class="Bool (strict)"("Blinking"=TRUE ("Blinkend")) -> ()  [unwired: 2 in, 2 out]
                    n623 = invoke class="VI" method="Ctrl Val.Set"(reference=w684, error in=w681, "Control Name"="AutoClose", "Value"=TRUE ("Blinkend")) -> (reference out=w683:refnum<vi>, error out=w682:errorcluster)  [unwired: 1 in, 3 out]
                    n624 = invoke on="Invoke Node" class="VI" method="FP.Open"(reference=w683, error in=w682, "Activate"=TRUE ("Activate?")) -> (reference out=w699:refnum<vi>, error out=w698:errorcluster)  [unwired: 2 in, 3 out]
                    n625 = invoke on="Invoke Node" class="VI" method="Run VI"(reference=w699, error in=w698, "Wait until done"=FALSE ("Wait Until Done"), "Auto Dispose Ref"=TRUE ("Auto Dispose Reference")) -> ()  [unwired: 1 in, 5 out]
                  }
                }
              }
            }
          }
          event "Video Show": Value Change {
            n626 = event-data() -> ("NewVal"=w716:bool)  [unwired: 1 in, 4 out]
            n627 = case shown="True" w716 {
              frame False {
                n628 = call "Video Toolset Stop.vi"() -> ()  [unwired: 3 in]
              }
              frame True {
                n629 = local read "Snapshot Folder"() -> (w718:path)
                n630 = local read "Camera Name"() -> (w717:string)
                n631 = call "Video Toolset Start.vi"("Snapshot Folder"=w718, "Camera Name"=w717) -> ()  [unwired: 1 in]
              }
            }
          }
        }
      }
    }
    frame #3 {
      # "Close Connections"
      n632 = control-ref of="Dieses VI"() -> (w719:refnum<vi>)
      n633 = invoke class="VI" method="Default Vals.Reinit All"(reference=w719) -> ()  [unwired: 2 in, 3 out]
    }
  }
